vi "Client.vi"() -> ()   [LabVIEW 2020]
panel:
  out "Current Time":timestamp
  out "Login":bool
  in  "Tab Control":T1(tab)
  out "Status Word":string
  out "Status":bool
  in  "4":bool
  out "Pin Number":string
  in  "E":bool
  in  "0":bool
  in  "C":bool
  in  "9":bool
  in  "8":bool
  in  "7":bool
  in  "6":bool
  in  "5":bool
  in  "3":bool
  in  "2":bool
  in  "1":bool
  in  "Alarm System":bool
  in  "Door Automatically Open":bool
  in  "Holiday Mode":bool
  in  "Temperature(°C)":dbl(slide) scale=-20.0..50.0
  out "Temperature(°C)":dbl
  in  "Clock":timestamp
  in  "Master Curtain":bool
  in  "Master Door":bool
  in  "Master Light":bool
  in  "Living Area AirCon":bool
  in  "Brightness\n Porch Light":dbl(slide) scale=0.0..255.0
  in  "Brightness\nLiving Area Light 1":dbl(slide) scale=0.0..255.0
  in  "Brightness\nLiving Area Light 2":dbl(slide) scale=0.0..255.0
  in  "Porch Light":bool
  in  "Living Area Curtain":dbl(slide) scale=0.0..100.0
  in  "Main Door":bool
  in  "Volume":i32(knob) scale=0.0..100.0
  in  "Mute":bool
  in  "Fast Forward":bool
  in  "Fast Reverse":bool
  in  "Stop":bool
  in  "Pause":bool
  in  "Play":bool
  in  "On/Off":bool
  in  "Channel 2":bool
  in  "Channel 1":bool
  in  "Channel 3":bool
  in  "Channel 4":bool
  in  "Living Area Light 2":bool
  in  "Living Area Light 1":bool
  in  "Brightness\nLanai Light":dbl(slide) scale=0.0..255.0
  in  "Brightness\nDining Area Light 1":dbl(slide) scale=0.0..255.0
  in  "Brightness\nDining Area Light 2":dbl(slide) scale=0.0..255.0
  in  "Lanai Light":bool
  in  "Lanai Door":bool
  in  "Dining Area Light 2":bool
  in  "Dining Area Light 1":bool
  in  "Master Bedroom AirCon":bool
  in  "Brightness\nMaster Bedroom \nLight 1":dbl(slide) scale=0.0..255.0
  in  "Brightness\nMaster Bath \nLight":dbl(slide) scale=0.0..255.0
  in  "Brightness\nMaster Bedroom \nLight 2":dbl(slide) scale=0.0..255.0
  in  "Brightness\nMaster Bedroom \nW.I.C. Light":dbl(slide) scale=0.0..255.0
  in  "Master Bedroom Curtain":dbl(slide) scale=0.0..100.0
  in  "Master Bath Door":bool
  in  "Master Bedroom Door":bool
  in  "Master Bedroom W.I.C. Light":bool
  in  "Master Bath Light":bool
  in  "Master Bedroom Light 2":bool
  in  "Master Bedroom Light 1":bool
  in  "Bedroom 2 AirCon":bool
  in  "Brightness\nBedroom 2 \nLight 1":dbl(slide) scale=0.0..255.0
  in  "Brightness\nBedroom 2 \nLight 2":dbl(slide) scale=0.0..255.0
  in  "Brightness\nBedroom 2 \nW.I.C. Light":dbl(slide) scale=0.0..255.0
  in  "Bedroom 2 Curtain 2":dbl(slide) scale=0.0..100.0
  in  "Bedroom 2 Curtain 1":dbl(slide) scale=0.0..100.0
  in  "Bedroom 2 Door":bool
  in  "Bedroom 2 W.I.C. Light":bool
  in  "Bedroom 2 Light 2":bool
  in  "Bedroom 2 Light 1":bool
  in  "Bedroom 3 AirCon":bool
  in  "Brightness\nBedroom 3 \nLight 1":dbl(slide) scale=0.0..255.0
  in  "Brightness\nBedroom 3 \nLight 2":dbl(slide) scale=0.0..255.0
  in  "Bedroom 3 Curtain 2":dbl(slide) scale=0.0..100.0
  in  "Bedroom 3 Curtain 1":dbl(slide) scale=0.0..100.0
  in  "Bedroom 3 Door":bool
  in  "Bedroom 3 Light 2":bool
  in  "Bedroom 3 Light 1":bool
  in  "Brightness\nService Laundry \nLight 2":dbl(slide) scale=0.0..255.0
  in  "Brightness\nService Laundry \nLight 1":dbl(slide) scale=0.0..255.0
  in  "Service Laundry Light 1":bool
  in  "Service Laundry Light 2":bool
  in  "Service/Laundry Door":bool
  in  "Brightness\nT&B Light":dbl(slide) scale=0.0..255.0
  in  "Brightness\nKitchen \nLight 2":dbl(slide) scale=0.0..255.0
  in  "Brightness\nKitchen \nLight 1":dbl(slide) scale=0.0..255.0
  in  "Kitchen Curtain 2":dbl(slide) scale=0.0..100.0
  in  "Kitchen Curtain 1":dbl(slide) scale=0.0..100.0
  in  "T&B Door":bool
  in  "T&B Light":bool
  in  "Kitchen Light 2":bool
  in  "Kitchen Light 1":bool
  in  "Brightness\nGarage Light 1":dbl(slide) scale=0.0..255.0
  in  "Brightness\nGarage Light 2":dbl(slide) scale=0.0..255.0
  in  "Garage Light 2":bool
  in  "Garage Light 1":bool
  in  "Logout":bool
  # "Smart Home Control System"
  # "LOGIN PAGE"
  # "Main Control"
  # "Living Area"
  # "TV"
  # "Dining Area"
  # "Lanai"
  # "Lanai"
  # "Master Bedroom"
  # "Bedroom 2"
  # "Bedroom 3"
  # "Kitchen"
  # "Service / Laundry"
  # "Garage"
  # "Are you sure want to logout?"
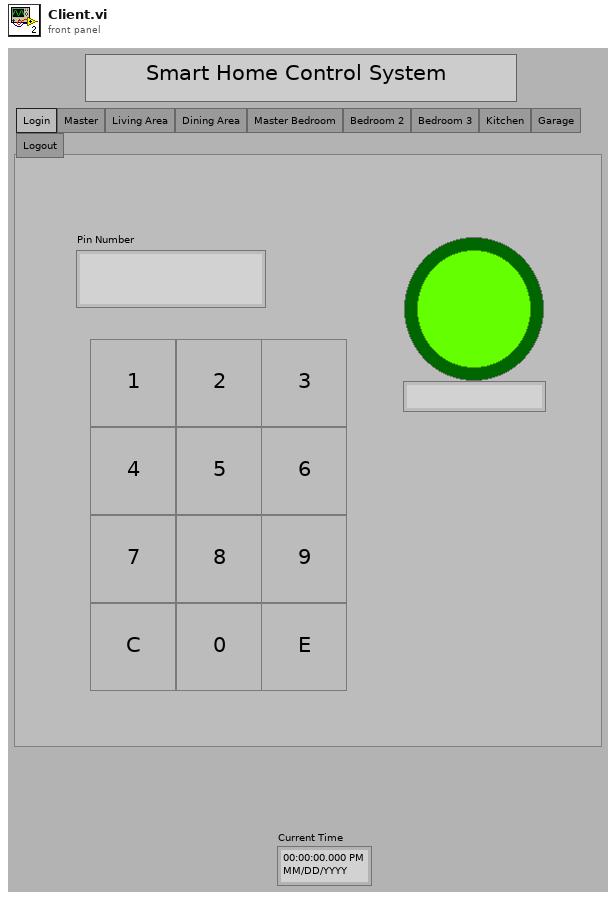
[diagram p1: front panel]
types:
  T1 = enum32{"Login", "Master", "Living Area", "Dining Area", "Master Bedroom", "Bedroom 2", "Bedroom 3", "Kitchen", "Garage", "Logout"}
  T2 = enum32{"Page Enabled", "Page Disabled", "Page Disabled & Grayed"}
  T3 = enum32{"Invalid", "Standard", "Closed", "Hidden", "Minimized", "Maximized"}
  T4 = typedef "LVDateTimeRec.ctl" = cluster{"fractional second":dbl, "second":i32, "minute":i32, "hour":i32, "day of month":i32, "month":i32, "year":i32, "day of week":i32, "day of year":i32, "DST":i32}
  T5 = enum8{"Enabled", "Disabled", "Disabled and Grayed Out"}
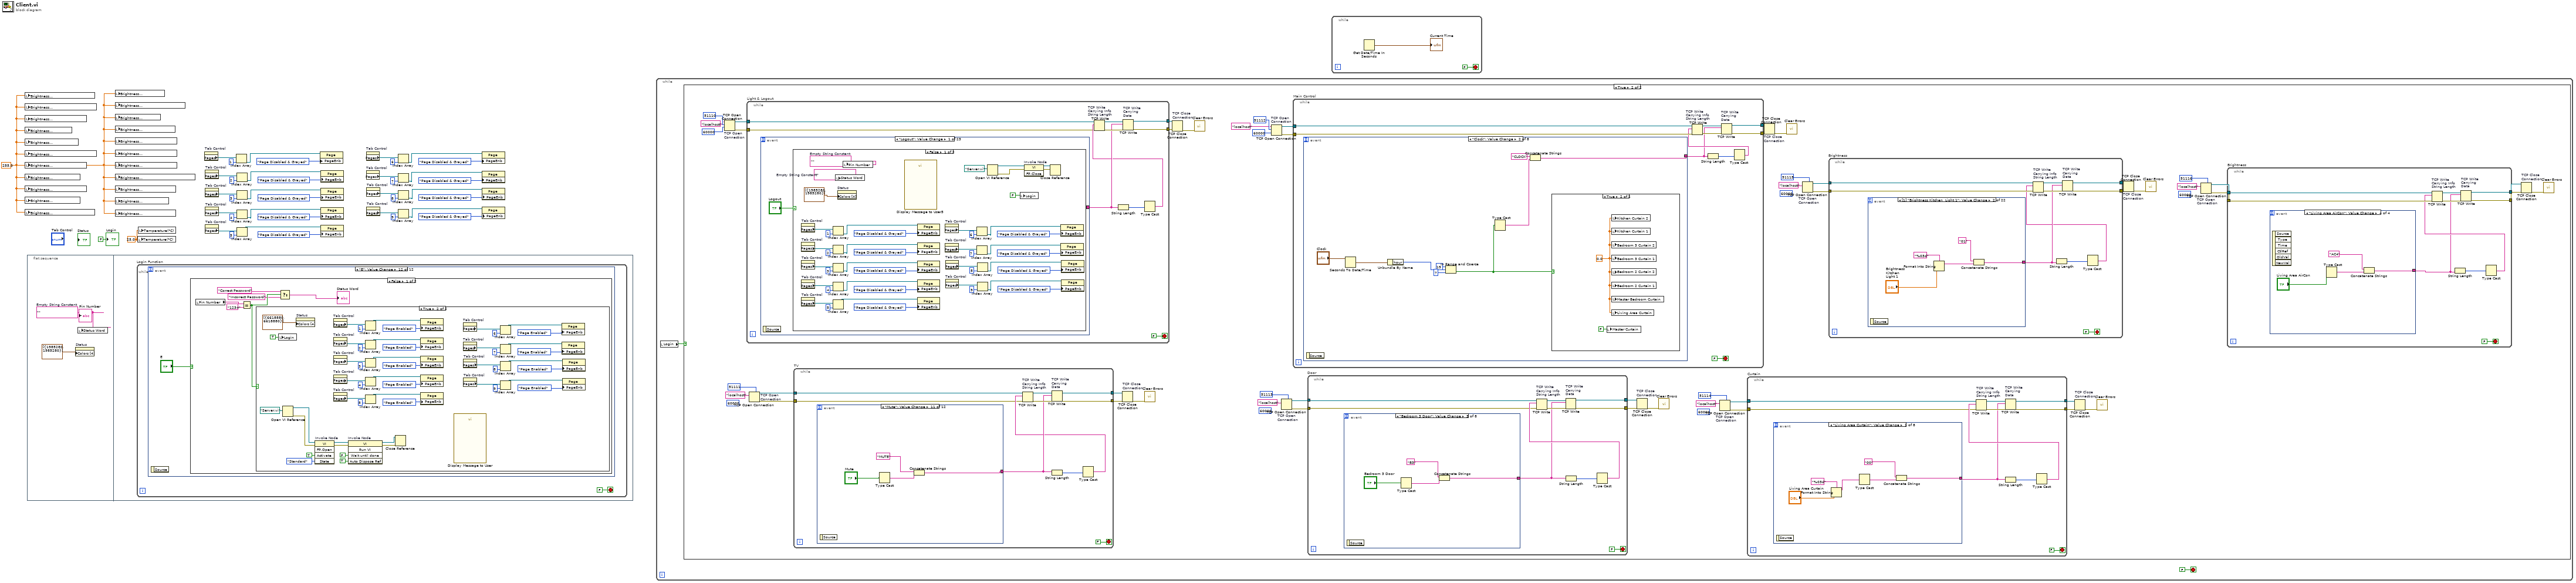
[diagram p0: block diagram]
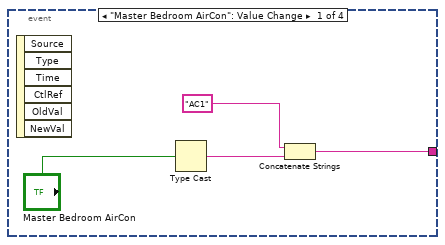
[diagram p3: hidden frame]
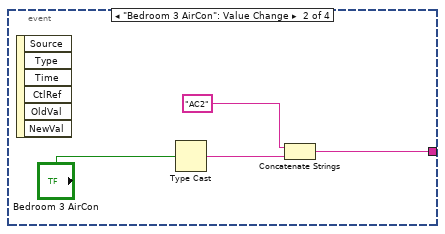
[diagram p4: hidden frame]
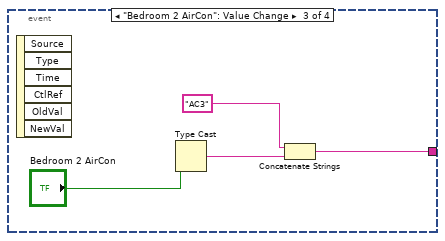
[diagram p5: hidden frame]
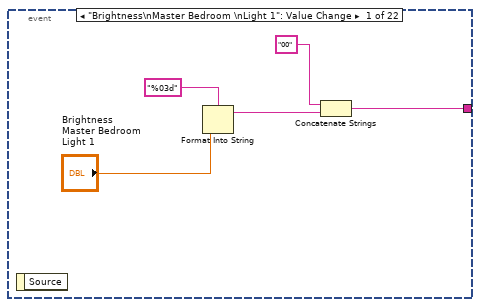
[diagram p6: hidden frame]
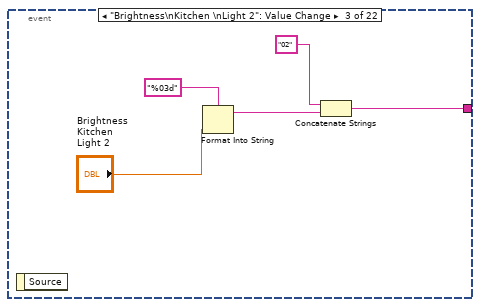
[diagram p7: hidden frame]
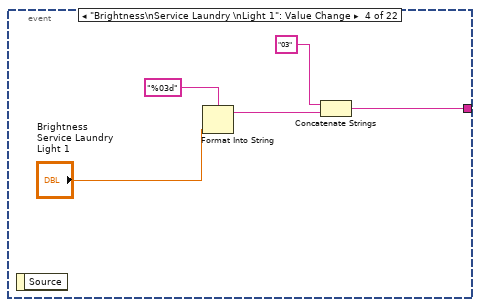
[diagram p8: hidden frame]
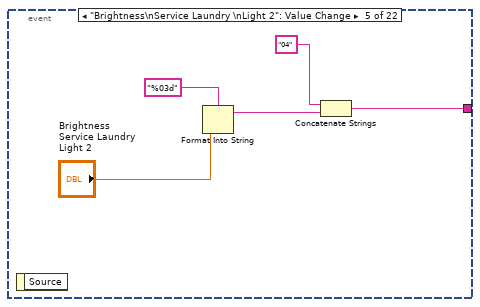
[diagram p9: hidden frame]
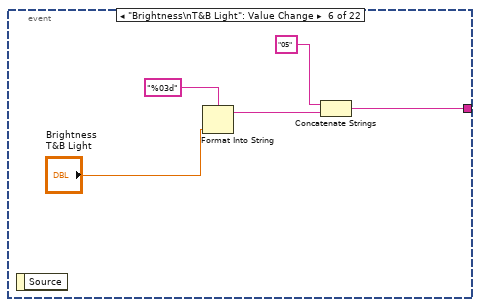
[diagram p10: hidden frame]
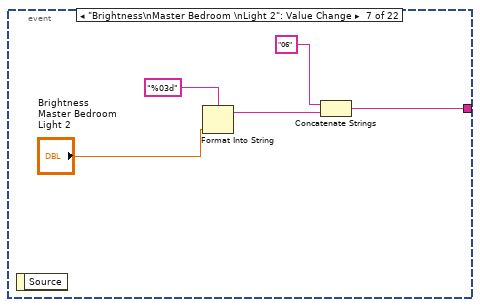
[diagram p11: hidden frame]
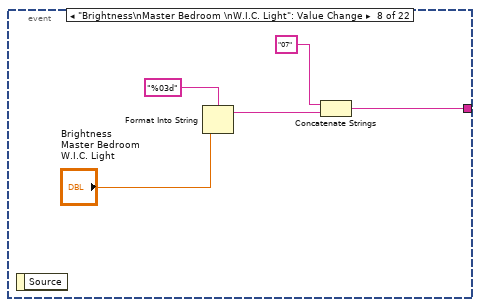
[diagram p12: hidden frame]
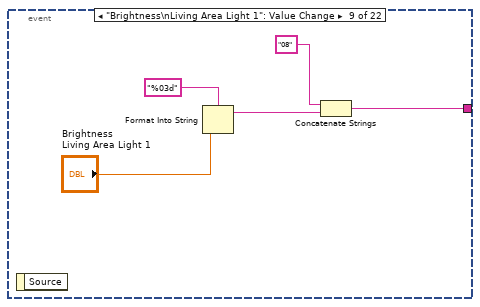
[diagram p13: hidden frame]
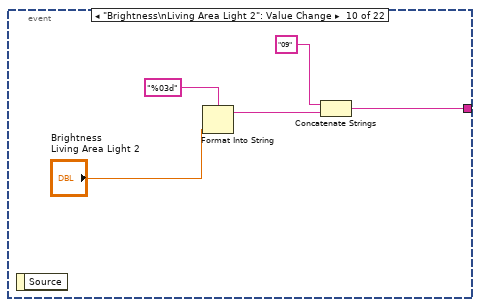
[diagram p14: hidden frame]
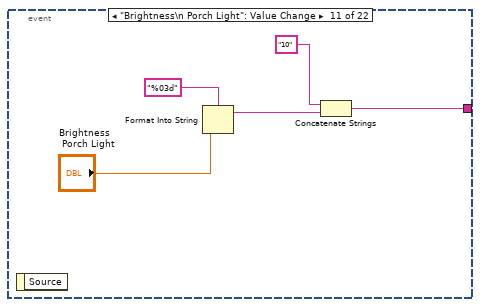
[diagram p15: hidden frame]
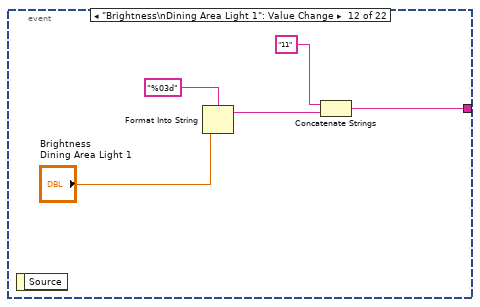
[diagram p16: hidden frame]
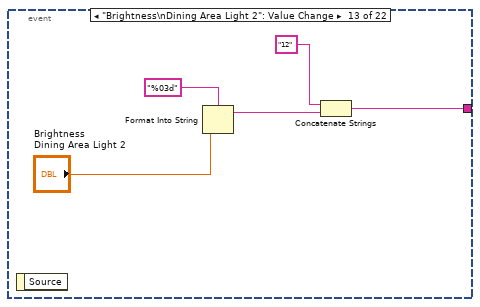
[diagram p17: hidden frame]
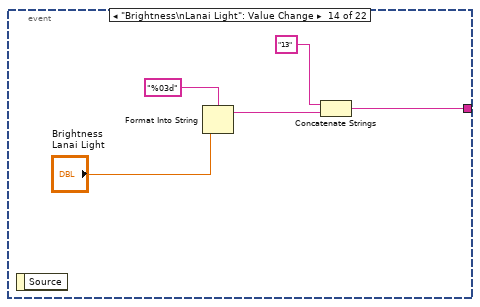
[diagram p18: hidden frame]
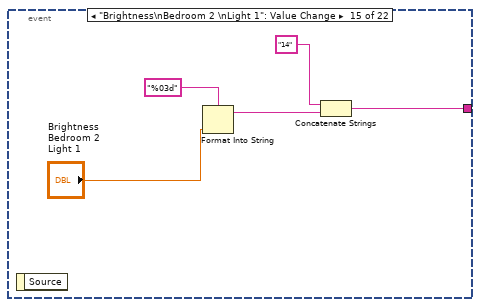
[diagram p19: hidden frame]
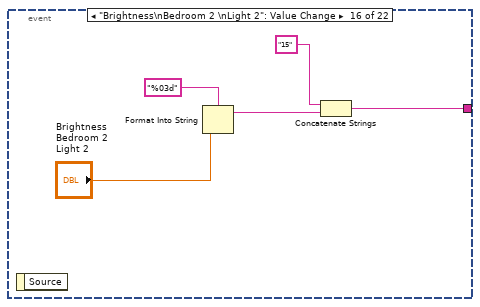
[diagram p20: hidden frame]
diagram:
  w1 = 255.0 ("Brightness\nBedroom 2 \nLight 1")
  w38 = 25.0 ("Temperature(°C)")
  n1 = local write "Brightness\nService Laundry \nLight 2"(w1) -> ()
  n2 = local write "Brightness\nMaster Bedroom \nLight 2"(w1) -> ()
  n3 = local write "Brightness\nDining Area Light 2"(w1) -> ()
  n4 = local write "Brightness\nLanai Light"(w1) -> ()
  n5 = local write "Brightness\nGarage Light 2"(w1) -> ()
  n6 = local write "Brightness\nMaster Bedroom \nLight 1"(w1) -> ()
  n7 = local write "Brightness\nBedroom 2 \nLight 1"(w1) -> ()
  n8 = local write "Brightness\nKitchen \nLight 1"(w1) -> ()
  n9 = local write "Brightness\nBedroom 2 \nLight 2"(w1) -> ()
  n10 = local write "Brightness\nKitchen \nLight 2"(w1) -> ()
  n11 = local write "Brightness\nBedroom 2 \nW.I.C. Light"(w1) -> ()
  n12 = flat-sequence {
    frame #0 {
      w40 = ""  # Empty String Constant
      n13 = property on="Status" class="Bool (strict)"("Colors [4]"=cluster{u32, u32}[] [{1985280, 1985280}]) -> ()  [unwired: 2 in, 2 out]
      n14 = local write "Status Word"(w40) -> ()
      "Pin Number" <- w40
    }
    frame #1 {
      n15 = while "Login Function" {
        stop <- FALSE stop-if-true
        n16 = event shown="[11] \"E\": Value Change" {
          selector: _ -> [_ _ _ _ _ _ _ _ _ _ _ _]
          dyn-events: _ -> [_ _ _ _ _ _ _ _ _ _ _ _]
          timeout: _ -> [_ _ _ _ _ _ _ _ _ _ _ _]
          event "1": Value Change {
            n17 = event-data() -> ()  [unwired: 1 in, 1 out]
            n18 = case shown="False" "1" {
              frame False {
                n19 = local read "Pin Number"() -> (w47:string)
                n20 = String Length "String \nLength"(string=w47) -> (length=w46:i32)
                n21 = Less?(x=w46, y=4) -> (x < y?=w44:bool)
                n22 = case shown="True" w44 {
                  frame False {
                  }
                  frame True {
                    n23 = local read "Pin Number"() -> (w50:string)
                    n24 = Concatenate Strings "Concatenate \nStrings"(w50, "1" ("string")) -> (w49:string)
                    n25 = local write "Pin Number"(w49) -> ()
                  }
                }
              }
              frame True {
              }
            }
          }
          event "2": Value Change {
            n26 = event-data() -> ()  [unwired: 1 in, 1 out]
            n27 = case shown="False" "2" {
              frame False {
                n28 = local read "Pin Number"() -> (w55:string)
                n29 = String Length "String \nLength"(string=w55) -> (length=w54:i32)
                n30 = Less?(x=w54, y=4) -> (x < y?=w52:bool)
                n31 = case shown="True" w52 {
                  frame False {
                  }
                  frame True {
                    n32 = local read "Pin Number"() -> (w58:string)
                    n33 = Concatenate Strings "Concatenate \nStrings"(w58, "2" ("string")) -> (w57:string)
                    n34 = local write "Pin Number"(w57) -> ()
                  }
                }
              }
              frame True {
              }
            }
          }
          event "3": Value Change {
            n35 = event-data() -> ()  [unwired: 1 in, 1 out]
            n36 = case shown="False" "3" {
              frame False {
                n37 = local read "Pin Number"() -> (w63:string)
                n38 = String Length "String \nLength"(string=w63) -> (length=w62:i32)
                n39 = Less?(x=w62, y=4) -> (x < y?=w60:bool)
                n40 = case shown="True" w60 {
                  frame False {
                  }
                  frame True {
                    n41 = local read "Pin Number"() -> (w66:string)
                    n42 = Concatenate Strings "Concatenate \nStrings"(w66, "3" ("string")) -> (w65:string)
                    n43 = local write "Pin Number"(w65) -> ()
                  }
                }
              }
              frame True {
              }
            }
          }
          event "4": Value Change {
            n44 = event-data() -> ()  [unwired: 1 in, 1 out]
            n45 = case shown="False" "4" {
              frame False {
                n46 = local read "Pin Number"() -> (w71:string)
                n47 = String Length "String \nLength"(string=w71) -> (length=w70:i32)
                n48 = Less?(x=w70, y=4) -> (x < y?=w68:bool)
                n49 = case shown="True" w68 {
                  frame False {
                  }
                  frame True {
                    n50 = local read "Pin Number"() -> (w74:string)
                    n51 = Concatenate Strings "Concatenate \nStrings"(w74, "4" ("string")) -> (w73:string)
                    n52 = local write "Pin Number"(w73) -> ()
                  }
                }
              }
              frame True {
              }
            }
          }
          event "5": Value Change {
            n53 = event-data() -> ()  [unwired: 1 in, 1 out]
            n54 = case shown="False" "5" {
              frame False {
                n55 = local read "Pin Number"() -> (w79:string)
                n56 = String Length "String \nLength"(string=w79) -> (length=w78:i32)
                n57 = Less?(x=w78, y=4) -> (x < y?=w76:bool)
                n58 = case shown="True" w76 {
                  frame False {
                  }
                  frame True {
                    n59 = local read "Pin Number"() -> (w82:string)
                    n60 = Concatenate Strings "Concatenate \nStrings"(w82, "5" ("string")) -> (w81:string)
                    n61 = local write "Pin Number"(w81) -> ()
                  }
                }
              }
              frame True {
              }
            }
          }
          event "6": Value Change {
            n62 = event-data() -> ()  [unwired: 1 in, 1 out]
            n63 = case shown="False" "6" {
              frame False {
                n64 = local read "Pin Number"() -> (w87:string)
                n65 = String Length "String \nLength"(string=w87) -> (length=w86:i32)
                n66 = Less?(x=w86, y=4) -> (x < y?=w84:bool)
                n67 = case shown="True" w84 {
                  frame False {
                  }
                  frame True {
                    n68 = local read "Pin Number"() -> (w90:string)
                    n69 = Concatenate Strings "Concatenate \nStrings"(w90, "6" ("string")) -> (w89:string)
                    n70 = local write "Pin Number"(w89) -> ()
                  }
                }
              }
              frame True {
              }
            }
          }
          event "7": Value Change {
            n71 = event-data() -> ()  [unwired: 1 in, 1 out]
            n72 = case shown="False" "7" {
              frame False {
                n73 = local read "Pin Number"() -> (w95:string)
                n74 = String Length "String \nLength"(string=w95) -> (length=w94:i32)
                n75 = Less?(x=w94, y=4) -> (x < y?=w92:bool)
                n76 = case shown="True" w92 {
                  frame False {
                  }
                  frame True {
                    n77 = local read "Pin Number"() -> (w98:string)
                    n78 = Concatenate Strings "Concatenate \nStrings"(w98, "7" ("string")) -> (w97:string)
                    n79 = local write "Pin Number"(w97) -> ()
                  }
                }
              }
              frame True {
              }
            }
          }
          event "8": Value Change {
            n80 = event-data() -> ()  [unwired: 1 in, 1 out]
            n81 = case shown="False" "8" {
              frame False {
                n82 = local read "Pin Number"() -> (w103:string)
                n83 = String Length "String \nLength"(string=w103) -> (length=w102:i32)
                n84 = Less?(x=w102, y=4) -> (x < y?=w100:bool)
                n85 = case shown="True" w100 {
                  frame False {
                  }
                  frame True {
                    n86 = local read "Pin Number"() -> (w106:string)
                    n87 = Concatenate Strings "Concatenate \nStrings"(w106, "8" ("string")) -> (w105:string)
                    n88 = local write "Pin Number"(w105) -> ()
                  }
                }
              }
              frame True {
              }
            }
          }
          event "9": Value Change {
            n89 = event-data() -> ()  [unwired: 1 in, 1 out]
            n90 = case shown="False" "9" {
              frame False {
                n91 = local read "Pin Number"() -> (w111:string)
                n92 = String Length "String \nLength"(string=w111) -> (length=w110:i32)
                n93 = Less?(x=w110, y=4) -> (x < y?=w108:bool)
                n94 = case shown="True" w108 {
                  frame False {
                  }
                  frame True {
                    n95 = local read "Pin Number"() -> (w114:string)
                    n96 = Concatenate Strings "Concatenate \nStrings"(w114, "9" ("string")) -> (w113:string)
                    n97 = local write "Pin Number"(w113) -> ()
                  }
                }
              }
              frame True {
              }
            }
          }
          event "0": Value Change {
            n98 = event-data() -> ()  [unwired: 1 in, 1 out]
            n99 = case shown="False" "0" {
              frame False {
                n100 = local read "Pin Number"() -> (w119:string)
                n101 = String Length "String \nLength"(string=w119) -> (length=w118:i32)
                n102 = Less?(x=w118, y=4) -> (x < y?=w116:bool)
                n103 = case shown="True" w116 {
                  frame False {
                  }
                  frame True {
                    n104 = local read "Pin Number"() -> (w122:string)
                    n105 = Concatenate Strings "Concatenate \nStrings"(w122, "0" ("string")) -> (w121:string)
                    n106 = local write "Pin Number"(w121) -> ()
                  }
                }
              }
              frame True {
              }
            }
          }
          event "C": Value Change {
            n107 = event-data() -> ()  [unwired: 1 in, 1 out]
            n108 = case shown="False" "C" {
              frame False {
                w124 = ""  # Empty String Constant
                n109 = local write "Pin Number"(w124) -> ()
              }
              frame True {
              }
            }
          }
          event "E": Value Change {
            n110 = event-data() -> ()  [unwired: 1 in, 1 out]
            n111 = case shown="False" "E" {
              frame False {
                n112 = local read "Pin Number"() -> (w131:string)
                n113 = Equal?(x=w131, y="1234") -> (x = y?=w129:bool)
                n114 = case shown="True" w129 {
                  frame False {
                    n115 = property on="Status" class="Bool (strict)"("Colors [4]"=cluster{u32, u32}[] [{16713728, 16714752}]) -> ()  [unwired: 2 in, 2 out]
                  }
                  frame True {
                    n116 = local write "Login"(TRUE ("Login")) -> ()
                    n117 = Open VI Reference(vi path=path "Server.vi") -> (vi reference=w179:refnum<vi>, error out=w178:errorcluster)  [unwired: 5 in]
                    n118 = property on="Status" class="Bool (strict)"("Colors [4]"=cluster{u32, u32}[] [{6618880, 6618880}]) -> ()  [unwired: 2 in, 2 out]
                    n119 = invoke on="Invoke Node" class="VI" method="FP.Open"(reference=w179, error in=w178, "Activate"=TRUE ("Activate?"), "State"=T3."Standard") -> (reference out=w173:refnum<vi>, error out=w172:errorcluster)  [unwired: 1 in, 3 out]
                    n120 = property on="Tab Control" class="TabCtl (strict)"() -> ("Pages"=w163:refnum<vi>[])  [unwired: 2 in, 2 out]
                    n121 = property on="Tab Control" class="TabCtl (strict)"() -> ("Pages"=w158:refnum<vi>[])  [unwired: 2 in, 2 out]
                    n122 = property on="Tab Control" class="TabCtl (strict)"() -> ("Pages"=w150:refnum<vi>[])  [unwired: 2 in, 2 out]
                    n123 = property on="Tab Control" class="TabCtl (strict)"() -> ("Pages"=w155:refnum<vi>[])  [unwired: 2 in, 2 out]
                    n124 = property on="Tab Control" class="TabCtl (strict)"() -> ("Pages"=w166:refnum<vi>[])  [unwired: 2 in, 2 out]
                    n125 = invoke on="Invoke Node" class="VI" method="Run VI"(reference=w173, error in=w172, "Wait until done"=FALSE ("Wait Until Done"), "Auto Dispose Ref"=TRUE ("Auto Dispose Reference")) -> (reference out=w171:refnum<vi>, error out=w170:errorcluster)  [unwired: 1 in, 3 out]
                    n126 = Index Array "Index Array"(array=w163, index=1) -> (element=w162:refnum<vi>)
                    n127 = Index Array "Index Array"(array=w158, index=2) -> (element=w159:refnum<vi>)
                    n128 = Index Array "Index Array"(array=w150, index=3) -> (element=w151:refnum<vi>)
                    n129 = Index Array "Index Array"(array=w155, index=4) -> (element=w154:refnum<vi>)
                    n130 = Index Array "Index Array"(array=w166, index=5) -> (element=w168:refnum<vi>)
                    n131 = Close Reference(reference=w171, error in (no error)=w170) -> ()  [unwired: 1 out]
                    n132 = property class="Page"(reference=w162, "PageEnb"=T2."Page Enabled" ("Page Enabled State")) -> ()  [unwired: 1 in, 2 out]
                    n133 = property class="Page"(reference=w159, "PageEnb"=T2."Page Enabled" ("Page Enabled State")) -> ()  [unwired: 1 in, 2 out]
                    n134 = property class="Page"(reference=w151, "PageEnb"=T2."Page Enabled" ("Page Enabled State")) -> ()  [unwired: 1 in, 2 out]
                    n135 = property class="Page"(reference=w154, "PageEnb"=T2."Page Enabled" ("Page Enabled State")) -> ()  [unwired: 1 in, 2 out]
                    n136 = property class="Page"(reference=w168, "PageEnb"=T2."Page Enabled" ("Page Enabled State")) -> ()  [unwired: 1 in, 2 out]
                    n137 = call "Display Message to User"() -> ()  [unwired: 10 in, 2 out]
                    n138 = property on="Tab Control" class="TabCtl (strict)"() -> ("Pages"=w141:refnum<vi>[])  [unwired: 2 in, 2 out]
                    n139 = property on="Tab Control" class="TabCtl (strict)"() -> ("Pages"=w144:refnum<vi>[])  [unwired: 2 in, 2 out]
                    n140 = property on="Tab Control" class="TabCtl (strict)"() -> ("Pages"=w148:refnum<vi>[])  [unwired: 2 in, 2 out]
                    n141 = property on="Tab Control" class="TabCtl (strict)"() -> ("Pages"=w145:refnum<vi>[])  [unwired: 2 in, 2 out]
                    n142 = Index Array "Index Array"(array=w141, index=6) -> (element=w142:refnum<vi>)
                    n143 = Index Array "Index Array"(array=w144, index=7) -> (element=w143:refnum<vi>)
                    n144 = Index Array "Index Array"(array=w148, index=8) -> (element=w147:refnum<vi>)
                    n145 = Index Array "Index Array"(array=w145, index=9) -> (element=w146:refnum<vi>)
                    n146 = property class="Page"(reference=w142, "PageEnb"=T2."Page Enabled" ("Page Enabled State")) -> ()  [unwired: 1 in, 2 out]
                    n147 = property class="Page"(reference=w143, "PageEnb"=T2."Page Enabled" ("Page Enabled State")) -> ()  [unwired: 1 in, 2 out]
                    n148 = property class="Page"(reference=w147, "PageEnb"=T2."Page Enabled" ("Page Enabled State")) -> ()  [unwired: 1 in, 2 out]
                    n149 = property class="Page"(reference=w146, "PageEnb"=T2."Page Enabled" ("Page Enabled State")) -> ()  [unwired: 1 in, 2 out]
                  }
                }
                n150 = Select(t="Correct Password", s=w129, f="Incorrect Password") -> (s? t:f=→"Status Word":string)
              }
              frame True {
              }
            }
          }
        }
      }
    }
  }
  n151 = local write "Brightness\n Porch Light"(w1) -> ()
  n152 = local write "Brightness\nService Laundry \nLight 1"(w1) -> ()
  n153 = local write "Brightness\nT&B Light"(w1) -> ()
  n154 = local write "Brightness\nMaster Bath \nLight"(w1) -> ()
  n155 = local write "Brightness\nDining Area Light 1"(w1) -> ()
  n156 = local write "Brightness\nBedroom 3 \nLight 1"(w1) -> ()
  n157 = local write "Brightness\nBedroom 3 \nLight 2"(w1) -> ()
  n158 = local write "Brightness\nMaster Bedroom \nW.I.C. Light"(w1) -> ()
  n159 = local write "Brightness\nLiving Area Light 1"(w1) -> ()
  n160 = local write "Brightness\nGarage Light 1"(w1) -> ()
  n161 = local write "Brightness\nLiving Area Light 2"(w1) -> ()
  n162 = local write "Temperature(°C)"(w38) -> ()
  n163 = local write "Temperature(°C)"(w38) -> ()
  n164 = property on="Tab Control" class="TabCtl (strict)"() -> ("Pages"=w7:refnum<vi>[])  [unwired: 2 in, 2 out]
  n165 = property on="Tab Control" class="TabCtl (strict)"() -> ("Pages"=w12:refnum<vi>[])  [unwired: 2 in, 2 out]
  n166 = property on="Tab Control" class="TabCtl (strict)"() -> ("Pages"=w20:refnum<vi>[])  [unwired: 2 in, 2 out]
  n167 = property on="Tab Control" class="TabCtl (strict)"() -> ("Pages"=w15:refnum<vi>[])  [unwired: 2 in, 2 out]
  n168 = property on="Tab Control" class="TabCtl (strict)"() -> ("Pages"=w4:refnum<vi>[])  [unwired: 2 in, 2 out]
  n169 = Index Array "Index Array"(array=w7, index=1) -> (element=w8:refnum<vi>)
  n170 = Index Array "Index Array"(array=w12, index=2) -> (element=w11:refnum<vi>)
  n171 = Index Array "Index Array"(array=w20, index=3) -> (element=w19:refnum<vi>)
  n172 = Index Array "Index Array"(array=w15, index=4) -> (element=w16:refnum<vi>)
  n173 = Index Array "Index Array"(array=w4, index=5) -> (element=w2:refnum<vi>)
  n174 = property class="Page"(reference=w8, "PageEnb"=T2."Page Disabled & Grayed" ("Page Enabled State")) -> ()  [unwired: 1 in, 2 out]
  n175 = property class="Page"(reference=w11, "PageEnb"=T2."Page Disabled & Grayed" ("Page Enabled State")) -> ()  [unwired: 1 in, 2 out]
  n176 = property class="Page"(reference=w19, "PageEnb"=T2."Page Disabled & Grayed" ("Page Enabled State")) -> ()  [unwired: 1 in, 2 out]
  n177 = property class="Page"(reference=w16, "PageEnb"=T2."Page Disabled & Grayed" ("Page Enabled State")) -> ()  [unwired: 1 in, 2 out]
  n178 = property class="Page"(reference=w2, "PageEnb"=T2."Page Disabled & Grayed" ("Page Enabled State")) -> ()  [unwired: 1 in, 2 out]
  n179 = property on="Tab Control" class="TabCtl (strict)"() -> ("Pages"=w36:refnum<vi>[])  [unwired: 2 in, 2 out]
  n180 = property on="Tab Control" class="TabCtl (strict)"() -> ("Pages"=w31:refnum<vi>[])  [unwired: 2 in, 2 out]
  n181 = property on="Tab Control" class="TabCtl (strict)"() -> ("Pages"=w23:refnum<vi>[])  [unwired: 2 in, 2 out]
  n182 = property on="Tab Control" class="TabCtl (strict)"() -> ("Pages"=w28:refnum<vi>[])  [unwired: 2 in, 2 out]
  n183 = Index Array "Index Array"(array=w36, index=6) -> (element=w35:refnum<vi>)
  n184 = Index Array "Index Array"(array=w31, index=7) -> (element=w32:refnum<vi>)
  n185 = Index Array "Index Array"(array=w23, index=8) -> (element=w24:refnum<vi>)
  n186 = Index Array "Index Array"(array=w28, index=9) -> (element=w27:refnum<vi>)
  n187 = property class="Page"(reference=w35, "PageEnb"=T2."Page Disabled & Grayed" ("Page Enabled State")) -> ()  [unwired: 1 in, 2 out]
  n188 = property class="Page"(reference=w32, "PageEnb"=T2."Page Disabled & Grayed" ("Page Enabled State")) -> ()  [unwired: 1 in, 2 out]
  n189 = property class="Page"(reference=w24, "PageEnb"=T2."Page Disabled & Grayed" ("Page Enabled State")) -> ()  [unwired: 1 in, 2 out]
  n190 = property class="Page"(reference=w27, "PageEnb"=T2."Page Disabled & Grayed" ("Page Enabled State")) -> ()  [unwired: 1 in, 2 out]
  n191 = while {
    stop <- FALSE stop-if-true
    n192 = local read "Login"() -> (w183:bool)
    n193 = case shown="True" w183 {
      frame False {
      }
      frame True {
        (unwired) 60000 ("timeout ms (60000)")
        (unwired) 60000 ("timeout ms (60000)")
        (unwired) 60000 ("timeout ms (60000)")
        (unwired) 60000 ("timeout ms (60000)")
        (unwired) 60000 ("timeout ms (60000)")
        n194 = TCP Open Connection "TCP Open \nConnection"(address="localhost", remote port or service name=u16 51110, timeout ms (60000)=60000) -> (connection ID=w230:refnum<k5>, error out=w231:errorcluster)  [unwired: 2 in]
        n195 = while "Light & Logout" {
          tunnel: w231 -> [w614]
          tunnel: w230 -> [w613]
          tunnel: [w612] -> w228
          tunnel: [w611] -> w227
          stop <- FALSE stop-if-true
          n196 = event shown="[0] \"Logout\": Value Change" {
            selector: _ -> [_ _ _ _ _ _ _ _ _ _ _ _ _ _ _ _ _ _ _ _ _ _ _]
            dyn-events: _ -> [_ _ _ _ _ _ _ _ _ _ _ _ _ _ _ _ _ _ _ _ _ _ _]
            timeout: _ -> [_ _ _ _ _ _ _ _ _ _ _ _ _ _ _ _ _ _ _ _ _ _ _]
            tunnel: [_ w666 w671 w675 w679 w683 w687 w691 w695 w699 w703 w707 w711 w715 w719 w723 w727 w731 w735 w739 w743 w747 w751] -> w617
            event "Logout": Value Change {
              n197 = event-data() -> ()  [unwired: 1 in, 1 out]
              n198 = case shown="False" "Logout" {
                frame False {
                  w659 = ""  # Empty String Constant
                  w657 = ""  # Empty String Constant
                  n199 = property on="Tab Control" class="TabCtl (strict)"() -> ("Pages"=w641:refnum<vi>[])  [unwired: 2 in, 2 out]
                  n200 = property on="Tab Control" class="TabCtl (strict)"() -> ("Pages"=w644:refnum<vi>[])  [unwired: 2 in, 2 out]
                  n201 = property on="Tab Control" class="TabCtl (strict)"() -> ("Pages"=w648:refnum<vi>[])  [unwired: 2 in, 2 out]
                  n202 = property on="Tab Control" class="TabCtl (strict)"() -> ("Pages"=w645:refnum<vi>[])  [unwired: 2 in, 2 out]
                  n203 = property on="Tab Control" class="TabCtl (strict)"() -> ("Pages"=w640:refnum<vi>[])  [unwired: 2 in, 2 out]
                  n204 = Index Array "Index Array"(array=w641, index=1) -> (element=w642:refnum<vi>)
                  n205 = Index Array "Index Array"(array=w644, index=2) -> (element=w643:refnum<vi>)
                  n206 = Index Array "Index Array"(array=w648, index=3) -> (element=w647:refnum<vi>)
                  n207 = Index Array "Index Array"(array=w645, index=4) -> (element=w646:refnum<vi>)
                  n208 = Index Array "Index Array"(array=w640, index=5) -> (element=w639:refnum<vi>)
                  n209 = local write "Status Word"(w657) -> ()
                  n210 = property on="Status" class="Bool (strict)"("Colors [4]"=cluster{u32, u32}[] [{1985280, 1985280}]) -> ()  [unwired: 2 in, 2 out]
                  n211 = local write "Pin Number"(w659) -> ()
                  n212 = call "Display Message to User3"() -> ()  [unwired: 10 in, 2 out]
                  n213 = property class="Page"(reference=w642, "PageEnb"=T2."Page Disabled & Grayed" ("Page Enabled State")) -> ()  [unwired: 1 in, 2 out]
                  n214 = property class="Page"(reference=w643, "PageEnb"=T2."Page Disabled & Grayed" ("Page Enabled State")) -> ()  [unwired: 1 in, 2 out]
                  n215 = property class="Page"(reference=w647, "PageEnb"=T2."Page Disabled & Grayed" ("Page Enabled State")) -> ()  [unwired: 1 in, 2 out]
                  n216 = property class="Page"(reference=w646, "PageEnb"=T2."Page Disabled & Grayed" ("Page Enabled State")) -> ()  [unwired: 1 in, 2 out]
                  n217 = property class="Page"(reference=w639, "PageEnb"=T2."Page Disabled & Grayed" ("Page Enabled State")) -> ()  [unwired: 1 in, 2 out]
                  n218 = property on="Tab Control" class="TabCtl (strict)"() -> ("Pages"=w656:refnum<vi>[])  [unwired: 2 in, 2 out]
                  n219 = property on="Tab Control" class="TabCtl (strict)"() -> ("Pages"=w653:refnum<vi>[])  [unwired: 2 in, 2 out]
                  n220 = property on="Tab Control" class="TabCtl (strict)"() -> ("Pages"=w649:refnum<vi>[])  [unwired: 2 in, 2 out]
                  n221 = property on="Tab Control" class="TabCtl (strict)"() -> ("Pages"=w652:refnum<vi>[])  [unwired: 2 in, 2 out]
                  n222 = Index Array "Index Array"(array=w656, index=6) -> (element=w655:refnum<vi>)
                  n223 = Index Array "Index Array"(array=w653, index=7) -> (element=w654:refnum<vi>)
                  n224 = Index Array "Index Array"(array=w649, index=8) -> (element=w650:refnum<vi>)
                  n225 = Index Array "Index Array"(array=w652, index=9) -> (element=w651:refnum<vi>)
                  n226 = Open VI Reference(vi path=path "Server.vi") -> (vi reference=w664:refnum<vi>, error out=w665:errorcluster)  [unwired: 5 in]
                  n227 = local write "Login"(FALSE ("Status 2")) -> ()
                  n228 = invoke on="Invoke Node" class="VI" method="FP.Close"(reference=w664, error in=w665) -> (reference out=w663:refnum<vi>, error out=w662:errorcluster)  [unwired: 1 in, 1 out]
                  n229 = Close Reference(reference=w663, error in (no error)=w662) -> ()  [unwired: 1 out]
                  n230 = property class="Page"(reference=w655, "PageEnb"=T2."Page Disabled & Grayed" ("Page Enabled State")) -> ()  [unwired: 1 in, 2 out]
                  n231 = property class="Page"(reference=w654, "PageEnb"=T2."Page Disabled & Grayed" ("Page Enabled State")) -> ()  [unwired: 1 in, 2 out]
                  n232 = property class="Page"(reference=w650, "PageEnb"=T2."Page Disabled & Grayed" ("Page Enabled State")) -> ()  [unwired: 1 in, 2 out]
                  n233 = property class="Page"(reference=w651, "PageEnb"=T2."Page Disabled & Grayed" ("Page Enabled State")) -> ()  [unwired: 1 in, 2 out]
                }
                frame True {
                }
              }
            }
            event "Porch Light": Value Change {
              n234 = event-data() -> ()  [unwired: 1 in, 1 out]
              n235 = case shown="True" "Porch Light" {
                tunnel: ["PL/F" "PL/T"] -> w666
                frame False {
                }
                frame True {
                }
              }
            }
            event "Living Area Light 1": Value Change {
              n236 = event-data() -> ()  [unwired: 1 in, 1 out]
              n237 = case shown="True" "Living Area Light 1" {
                tunnel: ["LAL1/F" "LAL1/T"] -> w671
                frame False {
                }
                frame True {
                }
              }
            }
            event "Living Area Light 2": Value Change {
              n238 = event-data() -> ()  [unwired: 1 in, 1 out]
              n239 = case shown="True" "Living Area Light 2" {
                tunnel: ["LAL2/F" "LAL2/T"] -> w675
                frame False {
                }
                frame True {
                }
              }
            }
            event "Dining Area Light 1": Value Change {
              n240 = event-data() -> ()  [unwired: 1 in, 1 out]
              n241 = case shown="True" "Dining Area Light 1" {
                tunnel: ["DAL1/F" "DAL1/T"] -> w679
                frame False {
                }
                frame True {
                }
              }
            }
            event "Dining Area Light 2": Value Change {
              n242 = event-data() -> ()  [unwired: 1 in, 1 out]
              n243 = case shown="True" "Dining Area Light 2" {
                tunnel: ["DAL2/F" "DAL2/T"] -> w683
                frame False {
                }
                frame True {
                }
              }
            }
            event "Master Bedroom Light 1": Value Change {
              n244 = event-data() -> ()  [unwired: 1 in, 1 out]
              n245 = case shown="False" "Master Bedroom Light 1" {
                tunnel: ["MBL1/F" "MBL1/T"] -> w687
                frame False {
                }
                frame True {
                }
              }
            }
            event "Master Bedroom Light 2": Value Change {
              n246 = event-data() -> ()  [unwired: 1 in, 1 out]
              n247 = case shown="False" "Master Bedroom Light 2" {
                tunnel: ["MBL2/F" "MBL2/T"] -> w691
                frame False {
                }
                frame True {
                }
              }
            }
            event "Master Bath Light": Value Change {
              n248 = event-data() -> ()  [unwired: 1 in, 1 out]
              n249 = case shown="True" "Master Bath Light" {
                tunnel: ["MBL/F" "MBL/T"] -> w695
                frame False {
                }
                frame True {
                }
              }
            }
            event "Master Bedroom W.I.C. Light": Value Change {
              n250 = event-data() -> ()  [unwired: 1 in, 1 out]
              n251 = case shown="False" "Master Bedroom W.I.C. Light" {
                tunnel: ["MBWICL/F" "MBWICL/T"] -> w699
                frame False {
                }
                frame True {
                }
              }
            }
            event "Bedroom 2 Light 1": Value Change {
              n252 = event-data() -> ()  [unwired: 1 in, 1 out]
              n253 = case shown="False" "Bedroom 2 Light 1" {
                tunnel: ["B2L1/F" "B2L1/T"] -> w703
                frame False {
                }
                frame True {
                }
              }
            }
            event "Bedroom 2 Light 2": Value Change {
              n254 = event-data() -> ()  [unwired: 1 in, 1 out]
              n255 = case shown="False" "Bedroom 2 Light 2" {
                tunnel: ["B2L2/F" "B2L2/T"] -> w707
                frame False {
                }
                frame True {
                }
              }
            }
            event "Bedroom 2 W.I.C. Light": Value Change {
              n256 = event-data() -> ()  [unwired: 1 in, 1 out]
              n257 = case shown="False" "Bedroom 2 W.I.C. Light" {
                tunnel: ["B2WICL/F" "B2WICL/T"] -> w711
                frame False {
                }
                frame True {
                }
              }
            }
            event "Bedroom 3 Light 1": Value Change {
              n258 = event-data() -> ()  [unwired: 1 in, 1 out]
              n259 = case shown="False" "Bedroom 3 Light 1" {
                tunnel: ["B3L1/F" "B3L1/T"] -> w715
                frame False {
                }
                frame True {
                }
              }
            }
            event "Bedroom 3 Light 2": Value Change {
              n260 = event-data() -> ()  [unwired: 1 in, 1 out]
              n261 = case shown="False" "Bedroom 3 Light 2" {
                tunnel: ["B3L2/F" "B3L2/T"] -> w719
                frame False {
                }
                frame True {
                }
              }
            }
            event "Kitchen Light 1": Value Change {
              n262 = event-data() -> ()  [unwired: 1 in, 1 out]
              n263 = case shown="False" "Kitchen Light 1" {
                tunnel: ["KL1/F" "KL1/T"] -> w723
                frame False {
                }
                frame True {
                }
              }
            }
            event "Kitchen Light 2": Value Change {
              n264 = event-data() -> ()  [unwired: 1 in, 1 out]
              n265 = case shown="False" "Kitchen Light 2" {
                tunnel: ["KL2/F" "KL2/T"] -> w727
                frame False {
                }
                frame True {
                }
              }
            }
            event "T&B Light": Value Change {
              n266 = event-data() -> ()  [unwired: 1 in, 1 out]
              n267 = case shown="False" "T&B Light" {
                tunnel: ["TBL/F" "TBL/T"] -> w731
                frame False {
                }
                frame True {
                }
              }
            }
            event "Lanai Light": Value Change {
              n268 = event-data() -> ()  [unwired: 1 in, 1 out]
              n269 = case shown="False" "Lanai Light" {
                tunnel: ["LL/F" "LL/T"] -> w735
                frame False {
                }
                frame True {
                }
              }
            }
            event "Service Laundry Light 1": Value Change {
              n270 = event-data() -> ()  [unwired: 1 in, 1 out]
              n271 = case shown="False" "Service Laundry Light 1" {
                tunnel: ["SLL1/F" "SLL1/T"] -> w739
                frame False {
                }
                frame True {
                }
              }
            }
            event "Service Laundry Light 2": Value Change {
              n272 = event-data() -> ()  [unwired: 1 in, 1 out]
              n273 = case shown="False" "Service Laundry Light 2" {
                tunnel: ["SLL2/F" "SLL2/T"] -> w743
                frame False {
                }
                frame True {
                }
              }
            }
            event "Garage Light 1": Value Change {
              n274 = event-data() -> ()  [unwired: 1 in, 1 out]
              n275 = case shown="True" "Garage Light 1" {
                tunnel: ["GL1/F" "GL1/T"] -> w747
                frame False {
                }
                frame True {
                }
              }
            }
            event "Garage Light 2": Value Change {
              n276 = event-data() -> ()  [unwired: 1 in, 1 out]
              n277 = case shown="True" "Garage Light 2" {
                tunnel: ["GL2/F" "GL2/T"] -> w751
                frame False {
                }
                frame True {
                }
              }
            }
          }
          n278 = String Length(string=w617) -> (length=w616:i32)
          n279 = Type Cast(x=w616) -> (*(type *) &x=w615:string)  [unwired: 1 in]
          n280 = TCP Write "TCP Write\nCarrying Info\nString Length"(connection ID=w613, data in=w615, error in (no error)=w614) -> (connection ID out=w619:refnum<k5>, error out=w618:errorcluster)  [unwired: 1 in, 1 out]
          n281 = TCP Write "TCP Write\nCarrying\nData"(connection ID=w619, data in=w617, error in (no error)=w618) -> (connection ID out=w611:refnum<k5>, error out=w612:errorcluster)  [unwired: 1 in, 1 out]
        }
        n282 = TCP Open Connection "TCP Open \nConnection"(address="localhost", remote port or service name=u16 51111) -> (connection ID=w223:refnum<k5>, error out=w222:errorcluster)  [unwired: 3 in]
        n283 = while "TV" {
          tunnel: w222 -> [w585]
          tunnel: w223 -> [w584]
          tunnel: [w583] -> w225
          tunnel: [w582] -> w226
          stop <- FALSE stop-if-true
          n284 = event shown="[10] \"Mute\": Value Change" {
            selector: _ -> [_ _ _ _ _ _ _ _ _ _ _ _]
            dyn-events: _ -> [_ _ _ _ _ _ _ _ _ _ _ _]
            timeout: _ -> [_ _ _ _ _ _ _ _ _ _ _ _]
            tunnel: ["ONOF" ("string") "PLAY" ("string") "PAUS" ("string") "STOP" ("string") "FFWD" ("string") "FRWD" ("string") "C1" ("string") "C2" ("string") "C3" ("string") "C4" ("string") w602 w607] -> w588
            event "On/Off": Value Change {
              n285 = event-data() -> ()  [unwired: 1 in, 1 out]
            }
            event "Play": Value Change {
              n286 = event-data() -> ()  [unwired: 1 in, 1 out]
            }
            event "Pause": Value Change {
              n287 = event-data() -> ()  [unwired: 1 in, 1 out]
            }
            event "Stop": Value Change {
              n288 = event-data() -> ()  [unwired: 1 in, 1 out]
            }
            event "Fast Forward": Value Change {
              n289 = event-data() -> ()  [unwired: 1 in, 1 out]
            }
            event "Fast Reverse": Value Change {
              n290 = event-data() -> ()  [unwired: 1 in, 1 out]
            }
            event "Channel 1": Value Change {
              n291 = event-data() -> ()  [unwired: 1 in, 1 out]
            }
            event "Channel 2": Value Change {
              n292 = event-data() -> ()  [unwired: 1 in, 1 out]
            }
            event "Channel 3": Value Change {
              n293 = event-data() -> ()  [unwired: 1 in, 1 out]
            }
            event "Channel 4": Value Change {
              n294 = event-data() -> ()  [unwired: 1 in, 1 out]
            }
            event "Mute": Value Change {
              n295 = event-data() -> ()  [unwired: 1 in, 1 out]
              n296 = Type Cast(x="Mute") -> (*(type *) &x=w604:string)  [unwired: 1 in]
              n297 = Concatenate Strings "Concatenate Strings"("MUTE" ("string"), w604) -> (w602:string)
            }
            event "Volume": Value Change {
              n298 = event-data() -> ()  [unwired: 1 in, 1 out]
              n299 = Type Cast(x="Volume") -> (*(type *) &x=w609:string)  [unwired: 1 in]
              n300 = Concatenate Strings "Concatenate Strings"("VOLM" ("string"), w609) -> (w607:string)
            }
          }
          n301 = String Length(string=w588) -> (length=w589:i32)
          n302 = Type Cast(x=w589) -> (*(type *) &x=w587:string)  [unwired: 1 in]
          n303 = TCP Write "TCP Write\nCarrying Info\nString Length"(connection ID=w584, data in=w587, error in (no error)=w585) -> (connection ID out=w590:refnum<k5>, error out=w591:errorcluster)  [unwired: 1 in, 1 out]
          n304 = TCP Write "TCP Write\nCarrying\nData"(connection ID=w590, data in=w588, error in (no error)=w591) -> (connection ID out=w582:refnum<k5>, error out=w583:errorcluster)  [unwired: 1 in, 1 out]
        }
        n305 = TCP Close Connection "TCP Close \nConnection"(connection ID=w226, error in (no error)=w225) -> (error out=w224:errorcluster)  [unwired: 1 in, 1 out]
        n306 = call <vilib>:"Clear Errors.vi"("error in (no error)"=w224) -> ()  [unwired: 5 in, 2 out]
        n307 = TCP Close Connection "TCP Close \nConnection"(connection ID=w227, error in (no error)=w228) -> (error out=w229:errorcluster)  [unwired: 1 in, 1 out]
        n308 = call <vilib>:"Clear Errors.vi"("error in (no error)"=w229) -> ()  [unwired: 5 in, 2 out]
        n309 = TCP Open Connection "TCP Open \nConnection"(address="localhost", remote port or service name=u16 51112, timeout ms (60000)=60000) -> (connection ID=w215:refnum<k5>, error out=w219:errorcluster)  [unwired: 2 in]
        n310 = TCP Open Connection "TCP Open \nConnection"(address="localhost", remote port or service name=u16 51113) -> (connection ID=w208:refnum<k5>, error out=w207:errorcluster)  [unwired: 3 in]
        n311 = while "Main Control" {
          tunnel: w215 -> [w489]
          tunnel: [w487] -> w216
          tunnel: [w486] -> w217
          tunnel: w219 -> [w484]
          stop <- FALSE stop-if-true
          n312 = event shown="[1] \"Clock\": Value Change" {
            selector: _ -> [_ _ _ _ _ _ _ _]
            dyn-events: _ -> [_ _ _ _ _ _ _ _]
            timeout: _ -> [_ _ _ _ _ _ _ _]
            tunnel: [w503 w520 w526 w556 w561 w568 w572 w576] -> w481
            event "Temperature(°C)": Value Change {
              n313 = event-data() -> ()  [unwired: 1 in, 1 out]
              n314 = local read "Temperature(°C)"() -> (w499:dbl)
              n315 = local read "Temperature(°C)"() -> (w492:dbl)
              n316 = Greater?(x=w499, y=30.0) -> (0:w497:bool)
              n317 = Greater Or Equal?(x=w492, y=50.0) -> (x >= y?=w491:bool)
              n318 = case shown="True" w491 {
                frame False {
                }
                frame True {
                  w508 = 0.0 ("Bedroom 3 Curtain 1")
                  w509 = FALSE ("Main Door")
                  n319 = local write "Bedroom 2 Door"(w509) -> ()
                  n320 = local write "Bedroom 3 Door"(w509) -> ()
                  n321 = local write "Master Bedroom Door"(w509) -> ()
                  n322 = local write "Master Bath Door"(w509) -> ()
                  n323 = local write "Lanai Door"(w509) -> ()
                  n324 = local write "T&B Door"(w509) -> ()
                  n325 = local write "Service/Laundry Door"(w509) -> ()
                  n326 = local write "Main Door"(w509) -> ()
                  n327 = local write "Master Curtain"(FALSE ("Master Curtain")) -> ()
                  n328 = local write "Master Door"(TRUE ("Master Door")) -> ()
                  n329 = local write "Kitchen Curtain 2"(w508) -> ()
                  n330 = local write "Kitchen Curtain 1"(w508) -> ()
                  n331 = local write "Bedroom 3 Curtain 2"(w508) -> ()
                  n332 = local write "Bedroom 3 Curtain 1"(w508) -> ()
                  n333 = local write "Bedroom 2 Curtain 2"(w508) -> ()
                  n334 = local write "Bedroom 2 Curtain 1"(w508) -> ()
                  n335 = local write "Master Bedroom Curtain"(w508) -> ()
                  n336 = local write "Living Area Curtain"(w508) -> ()
                }
              }
              n337 = case shown="True" w497 {
                frame False {
                }
                frame True {
                  w511 = TRUE ("Bedroom 3 AirCon")
                  n338 = local write "Master Bedroom AirCon"(w511) -> ()
                  n339 = local write "Bedroom 3 AirCon"(w511) -> ()
                  n340 = local write "Bedroom 2 AirCon"(w511) -> ()
                  n341 = local write "Living Area AirCon"(w511) -> ()
                }
              }
              n342 = local read "Temperature(°C)"() -> (w502:dbl)
              n343 = local read "Temperature(°C)"() -> (w494:dbl)
              n344 = Format Into String "Format Into String"(format string="%02d", w502) -> (resulting string=w501:string)  [unwired: 2 in, 1 out]
              n345 = Concatenate Strings "Concatenate Strings"("TEMPE" ("string"), w501) -> (w503:string)
              n346 = Less?(x=w494, y=10.0) -> (x < y?=w496:bool)
              n347 = case shown="True" w496 {
                frame False {
                }
                frame True {
                  w510 = FALSE ("Bedroom 3 AirCon")
                  n348 = local write "Master Bedroom AirCon"(w510) -> ()
                  n349 = local write "Bedroom 3 AirCon"(w510) -> ()
                  n350 = local write "Bedroom 2 AirCon"(w510) -> ()
                  n351 = local write "Living Area AirCon"(w510) -> ()
                }
              }
              "Temperature(°C)" <- "Temperature(°C)"
            }
            event "Clock": Value Change {
              n352 = event-data() -> ()  [unwired: 1 in, 1 out]
              n353 = Seconds To Date/Time(time stamp (now)="Clock") -> (date time rec=w517:T4)  [unwired: 1 in]
              n354 = Unbundle By Name "Unbundle By Name"(w517) -> ("hour"=w516:i32)
              n355 = In Range and Coerce(upper limit=19, x=w516, lower limit=7) -> (In Range?=w512:bool)  [unwired: 1 out]
              n356 = Type Cast(x=w512) -> (*(type *) &x=w513:string)  [unwired: 1 in]
              n357 = Concatenate Strings "Concatenate Strings"("CLOCK" ("string"), w513) -> (w520:string)
              n358 = case shown="True" w512 {
                frame False {
                  w522 = 100.0 ("Bedroom 3 Curtain 1")
                  n359 = local write "Kitchen Curtain 2"(w522) -> ()
                  n360 = local write "Kitchen Curtain 1"(w522) -> ()
                  n361 = local write "Bedroom 3 Curtain 2"(w522) -> ()
                  n362 = local write "Bedroom 3 Curtain 1"(w522) -> ()
                  n363 = local write "Bedroom 2 Curtain 2"(w522) -> ()
                  n364 = local write "Bedroom 2 Curtain 1"(w522) -> ()
                  n365 = local write "Master Bedroom Curtain"(w522) -> ()
                  n366 = local write "Living Area Curtain"(w522) -> ()
                  n367 = local write "Master Curtain"(TRUE ("Master Curtain")) -> ()
                }
                frame True {
                  w524 = 0.0 ("Bedroom 3 Curtain 1")
                  n368 = local write "Master Curtain"(FALSE ("Master Curtain")) -> ()
                  n369 = local write "Kitchen Curtain 2"(w524) -> ()
                  n370 = local write "Kitchen Curtain 1"(w524) -> ()
                  n371 = local write "Bedroom 3 Curtain 2"(w524) -> ()
                  n372 = local write "Bedroom 3 Curtain 1"(w524) -> ()
                  n373 = local write "Bedroom 2 Curtain 2"(w524) -> ()
                  n374 = local write "Bedroom 2 Curtain 1"(w524) -> ()
                  n375 = local write "Master Bedroom Curtain"(w524) -> ()
                  n376 = local write "Living Area Curtain"(w524) -> ()
                }
              }
            }
            event "Master Light": Value Change {
              n377 = event-data() -> ()  [unwired: 1 in, 1 out]
              n378 = case shown="False" "Master Light" {
                frame False {
                  w529 = T5."Enabled" ("Disabled")
                  n379 = property on="Porch Light" class="Bool (strict)"("DisabledEnum"=w529) -> ()  [unwired: 2 in, 2 out]
                  n380 = property on="Living Area Light 1" class="Bool (strict)"("DisabledEnum"=w529) -> ()  [unwired: 2 in, 2 out]
                  n381 = property on="Living Area Light 2" class="Bool (strict)"("DisabledEnum"=w529) -> ()  [unwired: 2 in, 2 out]
                  n382 = property on="Dining Area Light 1" class="Bool (strict)"("DisabledEnum"=w529) -> ()  [unwired: 2 in, 2 out]
                  n383 = property on="Dining Area Light 2" class="Bool (strict)"("DisabledEnum"=w529) -> ()  [unwired: 2 in, 2 out]
                  n384 = property on="Master Bedroom Light 1" class="Bool (strict)"("DisabledEnum"=w529) -> ()  [unwired: 2 in, 2 out]
                  n385 = property on="Master Bedroom Light 2" class="Bool (strict)"("DisabledEnum"=w529) -> ()  [unwired: 2 in, 2 out]
                  n386 = property on="Master Bath Light" class="Bool (strict)"("DisabledEnum"=w529) -> ()  [unwired: 2 in, 2 out]
                  n387 = property on="Master Bedroom W.I.C. Light" class="Bool (strict)"("DisabledEnum"=w529) -> ()  [unwired: 2 in, 2 out]
                  n388 = property on="Bedroom 2 Light 1" class="Bool (strict)"("DisabledEnum"=w529) -> ()  [unwired: 2 in, 2 out]
                  n389 = property on="Bedroom 2 Light 2" class="Bool (strict)"("DisabledEnum"=w529) -> ()  [unwired: 2 in, 2 out]
                  n390 = property on="Bedroom 2 W.I.C. Light" class="Bool (strict)"("DisabledEnum"=w529) -> ()  [unwired: 2 in, 2 out]
                  n391 = property on="Bedroom 3 Light 1" class="Bool (strict)"("DisabledEnum"=w529) -> ()  [unwired: 2 in, 2 out]
                  n392 = property on="Bedroom 3 Light 2" class="Bool (strict)"("DisabledEnum"=w529) -> ()  [unwired: 2 in, 2 out]
                  n393 = property on="Kitchen Light 1" class="Bool (strict)"("DisabledEnum"=w529) -> ()  [unwired: 2 in, 2 out]
                  n394 = property on="Kitchen Light 2" class="Bool (strict)"("DisabledEnum"=w529) -> ()  [unwired: 2 in, 2 out]
                  n395 = property on="T&B Light" class="Bool (strict)"("DisabledEnum"=w529) -> ()  [unwired: 2 in, 2 out]
                  n396 = property on="Lanai Light" class="Bool (strict)"("DisabledEnum"=w529) -> ()  [unwired: 2 in, 2 out]
                  n397 = property on="Service Laundry Light 1" class="Bool (strict)"("DisabledEnum"=w529) -> ()  [unwired: 2 in, 2 out]
                  n398 = property on="Service Laundry Light 2" class="Bool (strict)"("DisabledEnum"=w529) -> ()  [unwired: 2 in, 2 out]
                  n399 = property on="Garage Light 2" class="Bool (strict)"("DisabledEnum"=w529) -> ()  [unwired: 2 in, 2 out]
                  n400 = property on="Garage Light 1" class="Bool (strict)"("DisabledEnum"=w529) -> ()  [unwired: 2 in, 2 out]
                }
                frame True {
                  n401 = flat-sequence {
                    frame #0 {
                      n402 = local write "Porch Light"(FALSE ("Porch Light")) -> ()
                      n403 = local write "Living Area Light 1"(FALSE ("Living Area Light 1")) -> ()
                      n404 = local write "Living Area Light 2"(FALSE ("Living Area Light 2")) -> ()
                      n405 = local write "Dining Area Light 1"(FALSE ("Dining Area Light 1")) -> ()
                      n406 = local write "Dining Area Light 2"(FALSE ("Dining Area Light 2")) -> ()
                      n407 = local write "Master Bedroom Light 1"(FALSE ("Master Bedroom Light 1")) -> ()
                      n408 = local write "Master Bedroom Light 2"(FALSE ("Master Bedroom Light 2")) -> ()
                      n409 = local write "Master Bath Light"(FALSE ("Master Bath Light")) -> ()
                      n410 = local write "Master Bedroom W.I.C. Light"(FALSE ("Master Bedroom W.I.C. Light")) -> ()
                      n411 = local write "Bedroom 2 Light 1"(FALSE ("Bedroom 2 Light 1")) -> ()
                      n412 = local write "Bedroom 2 Light 2"(FALSE ("Bedroom 2 Light 2")) -> ()
                      n413 = local write "Bedroom 2 W.I.C. Light"(FALSE ("Bedroom 2 W.I.C. Light")) -> ()
                      n414 = local write "Bedroom 3 Light 1"(FALSE ("Bedroom 3 Light 1")) -> ()
                      n415 = local write "Bedroom 3 Light 2"(FALSE ("Bedroom 3 Light 2")) -> ()
                      n416 = local write "Kitchen Light 1"(FALSE ("Kitchen Light 1")) -> ()
                      n417 = local write "Kitchen Light 2"(FALSE ("Kitchen Light 2")) -> ()
                      n418 = local write "T&B Light"(FALSE ("T&B Light")) -> ()
                      n419 = local write "Lanai Light"(FALSE ("Lanai Light")) -> ()
                      n420 = local write "Service Laundry Light 1"(FALSE ("Service Laundry Light 1")) -> ()
                      n421 = local write "Service Laundry Light 2"(FALSE ("Service Laundry Light 2")) -> ()
                      n422 = local write "Garage Light 1"(FALSE ("Garage Light 1")) -> ()
                      n423 = local write "Garage Light 2"(FALSE ("Garage Light 2")) -> ()
                    }
                    frame #1 {
                      w552 = T5."Disabled" ("Disabled")
                      n424 = property on="Porch Light" class="Bool (strict)"("DisabledEnum"=w552) -> ()  [unwired: 2 in, 2 out]
                      n425 = property on="Living Area Light 1" class="Bool (strict)"("DisabledEnum"=w552) -> ()  [unwired: 2 in, 2 out]
                      n426 = property on="Living Area Light 2" class="Bool (strict)"("DisabledEnum"=w552) -> ()  [unwired: 2 in, 2 out]
                      n427 = property on="Dining Area Light 1" class="Bool (strict)"("DisabledEnum"=w552) -> ()  [unwired: 2 in, 2 out]
                      n428 = property on="Dining Area Light 2" class="Bool (strict)"("DisabledEnum"=w552) -> ()  [unwired: 2 in, 2 out]
                      n429 = property on="Master Bedroom Light 1" class="Bool (strict)"("DisabledEnum"=w552) -> ()  [unwired: 2 in, 2 out]
                      n430 = property on="Master Bedroom Light 2" class="Bool (strict)"("DisabledEnum"=w552) -> ()  [unwired: 2 in, 2 out]
                      n431 = property on="Master Bath Light" class="Bool (strict)"("DisabledEnum"=w552) -> ()  [unwired: 2 in, 2 out]
                      n432 = property on="Master Bedroom W.I.C. Light" class="Bool (strict)"("DisabledEnum"=w552) -> ()  [unwired: 2 in, 2 out]
                      n433 = property on="Bedroom 2 Light 1" class="Bool (strict)"("DisabledEnum"=w552) -> ()  [unwired: 2 in, 2 out]
                      n434 = property on="Bedroom 2 Light 2" class="Bool (strict)"("DisabledEnum"=w552) -> ()  [unwired: 2 in, 2 out]
                      n435 = property on="Bedroom 2 W.I.C. Light" class="Bool (strict)"("DisabledEnum"=w552) -> ()  [unwired: 2 in, 2 out]
                      n436 = property on="Bedroom 3 Light 1" class="Bool (strict)"("DisabledEnum"=w552) -> ()  [unwired: 2 in, 2 out]
                      n437 = property on="Bedroom 3 Light 2" class="Bool (strict)"("DisabledEnum"=w552) -> ()  [unwired: 2 in, 2 out]
                      n438 = property on="Kitchen Light 1" class="Bool (strict)"("DisabledEnum"=w552) -> ()  [unwired: 2 in, 2 out]
                      n439 = property on="Kitchen Light 2" class="Bool (strict)"("DisabledEnum"=w552) -> ()  [unwired: 2 in, 2 out]
                      n440 = property on="T&B Light" class="Bool (strict)"("DisabledEnum"=w552) -> ()  [unwired: 2 in, 2 out]
                      n441 = property on="Lanai Light" class="Bool (strict)"("DisabledEnum"=w552) -> ()  [unwired: 2 in, 2 out]
                      n442 = property on="Service Laundry Light 1" class="Bool (strict)"("DisabledEnum"=w552) -> ()  [unwired: 2 in, 2 out]
                      n443 = property on="Service Laundry Light 2" class="Bool (strict)"("DisabledEnum"=w552) -> ()  [unwired: 2 in, 2 out]
                      n444 = property on="Garage Light 2" class="Bool (strict)"("DisabledEnum"=w552) -> ()  [unwired: 2 in, 2 out]
                      n445 = property on="Garage Light 1" class="Bool (strict)"("DisabledEnum"=w552) -> ()  [unwired: 2 in, 2 out]
                    }
                  }
                }
              }
              n446 = Type Cast(x="Master Light") -> (*(type *) &x=w528:string)  [unwired: 1 in]
              n447 = Concatenate Strings "Concatenate Strings"("MAINL" ("string"), w528) -> (w526:string)
            }
            event "Master Door": Value Change {
              n448 = event-data() -> ()  [unwired: 1 in, 1 out]
              n449 = case shown="True" "Master Door" {
                frame False {
                  w557 = T5."Enabled" ("Disabled")
                  n450 = property on="Main Door" class="Bool (strict)"("DisabledEnum"=w557) -> ()  [unwired: 2 in, 2 out]
                  n451 = property on="Bedroom 2 Door" class="Bool (strict)"("DisabledEnum"=w557) -> ()  [unwired: 2 in, 2 out]
                  n452 = property on="Bedroom 3 Door" class="Bool (strict)"("DisabledEnum"=w557) -> ()  [unwired: 2 in, 2 out]
                  n453 = property on="Master Bedroom Door" class="Bool (strict)"("DisabledEnum"=w557) -> ()  [unwired: 2 in, 2 out]
                  n454 = property on="Master Bath Door" class="Bool (strict)"("DisabledEnum"=w557) -> ()  [unwired: 2 in, 2 out]
                  n455 = property on="Lanai Door" class="Bool (strict)"("DisabledEnum"=w557) -> ()  [unwired: 2 in, 2 out]
                  n456 = property on="T&B Door" class="Bool (strict)"("DisabledEnum"=w557) -> ()  [unwired: 2 in, 2 out]
                  n457 = property on="Service/Laundry Door" class="Bool (strict)"("DisabledEnum"=w557) -> ()  [unwired: 2 in, 2 out]
                }
                frame True {
                  n458 = flat-sequence {
                    frame #0 {
                      w558 = FALSE ("Main Door")
                      n459 = local write "Bedroom 2 Door"(w558) -> ()
                      n460 = local write "Bedroom 3 Door"(w558) -> ()
                      n461 = local write "Master Bedroom Door"(w558) -> ()
                      n462 = local write "Master Bath Door"(w558) -> ()
                      n463 = local write "Lanai Door"(w558) -> ()
                      n464 = local write "T&B Door"(w558) -> ()
                      n465 = local write "Service/Laundry Door"(w558) -> ()
                      n466 = local write "Main Door"(w558) -> ()
                    }
                    frame #1 {
                      w559 = T5."Disabled" ("Disabled")
                      n467 = property on="Main Door" class="Bool (strict)"("DisabledEnum"=w559) -> ()  [unwired: 2 in, 2 out]
                      n468 = property on="Bedroom 2 Door" class="Bool (strict)"("DisabledEnum"=w559) -> ()  [unwired: 2 in, 2 out]
                      n469 = property on="Bedroom 3 Door" class="Bool (strict)"("DisabledEnum"=w559) -> ()  [unwired: 2 in, 2 out]
                      n470 = property on="Master Bedroom Door" class="Bool (strict)"("DisabledEnum"=w559) -> ()  [unwired: 2 in, 2 out]
                      n471 = property on="Master Bath Door" class="Bool (strict)"("DisabledEnum"=w559) -> ()  [unwired: 2 in, 2 out]
                      n472 = property on="Lanai Door" class="Bool (strict)"("DisabledEnum"=w559) -> ()  [unwired: 2 in, 2 out]
                      n473 = property on="T&B Door" class="Bool (strict)"("DisabledEnum"=w559) -> ()  [unwired: 2 in, 2 out]
                      n474 = property on="Service/Laundry Door" class="Bool (strict)"("DisabledEnum"=w559) -> ()  [unwired: 2 in, 2 out]
                    }
                  }
                }
              }
              n475 = Type Cast(x="Master Door") -> (*(type *) &x=w554:string)  [unwired: 1 in]
              n476 = Concatenate Strings "Concatenate Strings"("MAIND" ("string"), w554) -> (w556:string)
            }
            event "Master Curtain": Value Change {
              n477 = event-data() -> ()  [unwired: 1 in, 1 out]
              n478 = case shown="True" "Master Curtain" {
                frame False {
                  w564 = T5."Enabled" ("Disabled")
                  n479 = property on="Master Bedroom Curtain" class="Slide (strict)"("DisabledEnum"=w564) -> ()  [unwired: 2 in, 2 out]
                  n480 = property on="Living Area Curtain" class="Slide (strict)"("DisabledEnum"=w564) -> ()  [unwired: 2 in, 2 out]
                  n481 = property on="Kitchen Curtain 2" class="Slide (strict)"("DisabledEnum"=w564) -> ()  [unwired: 2 in, 2 out]
                  n482 = property on="Kitchen Curtain 1" class="Slide (strict)"("DisabledEnum"=w564) -> ()  [unwired: 2 in, 2 out]
                  n483 = property on="Bedroom 3 Curtain 2" class="Slide (strict)"("DisabledEnum"=w564) -> ()  [unwired: 2 in, 2 out]
                  n484 = property on="Bedroom 3 Curtain 1" class="Slide (strict)"("DisabledEnum"=w564) -> ()  [unwired: 2 in, 2 out]
                  n485 = property on="Bedroom 2 Curtain 2" class="Slide (strict)"("DisabledEnum"=w564) -> ()  [unwired: 2 in, 2 out]
                  n486 = property on="Bedroom 2 Curtain 1" class="Slide (strict)"("DisabledEnum"=w564) -> ()  [unwired: 2 in, 2 out]
                }
                frame True {
                  n487 = flat-sequence {
                    frame #0 {
                      w565 = 0.0 ("Bedroom 3 Curtain 1")
                      n488 = local write "Kitchen Curtain 2"(w565) -> ()
                      n489 = local write "Kitchen Curtain 1"(w565) -> ()
                      n490 = local write "Bedroom 3 Curtain 2"(w565) -> ()
                      n491 = local write "Bedroom 3 Curtain 1"(w565) -> ()
                      n492 = local write "Bedroom 2 Curtain 2"(w565) -> ()
                      n493 = local write "Bedroom 2 Curtain 1"(w565) -> ()
                      n494 = local write "Master Bedroom Curtain"(w565) -> ()
                      n495 = local write "Living Area Curtain"(w565) -> ()
                    }
                    frame #1 {
                      w566 = T5."Disabled" ("Disabled")
                      n496 = property on="Master Bedroom Curtain" class="Slide (strict)"("DisabledEnum"=w566) -> ()  [unwired: 2 in, 2 out]
                      n497 = property on="Living Area Curtain" class="Slide (strict)"("DisabledEnum"=w566) -> ()  [unwired: 2 in, 2 out]
                      n498 = property on="Kitchen Curtain 2" class="Slide (strict)"("DisabledEnum"=w566) -> ()  [unwired: 2 in, 2 out]
                      n499 = property on="Kitchen Curtain 1" class="Slide (strict)"("DisabledEnum"=w566) -> ()  [unwired: 2 in, 2 out]
                      n500 = property on="Bedroom 3 Curtain 2" class="Slide (strict)"("DisabledEnum"=w566) -> ()  [unwired: 2 in, 2 out]
                      n501 = property on="Bedroom 3 Curtain 1" class="Slide (strict)"("DisabledEnum"=w566) -> ()  [unwired: 2 in, 2 out]
                      n502 = property on="Bedroom 2 Curtain 2" class="Slide (strict)"("DisabledEnum"=w566) -> ()  [unwired: 2 in, 2 out]
                      n503 = property on="Bedroom 2 Curtain 1" class="Slide (strict)"("DisabledEnum"=w566) -> ()  [unwired: 2 in, 2 out]
                    }
                  }
                }
              }
              n504 = Type Cast(x="Master Curtain") -> (*(type *) &x=w563:string)  [unwired: 1 in]
              n505 = Concatenate Strings "Concatenate Strings"("MAINW" ("string"), w563) -> (w561:string)
            }
            event "Holiday Mode": Value Change {
              n506 = event-data() -> ()  [unwired: 1 in, 1 out]
              n507 = Type Cast(x="Holiday Mode") -> (*(type *) &x=w570:string)  [unwired: 1 in]
              n508 = Concatenate Strings "Concatenate Strings"("HLDMD" ("string"), w570) -> (w568:string)
            }
            event "Door Automatically Open": Value Change {
              n509 = event-data() -> ()  [unwired: 1 in, 1 out]
              n510 = Type Cast(x="Door Automatically Open") -> (*(type *) &x=w574:string)  [unwired: 1 in]
              n511 = Concatenate Strings "Concatenate Strings"("DRAOP" ("string"), w574) -> (w572:string)
            }
            event "Alarm System": Value Change {
              n512 = event-data() -> ()  [unwired: 1 in, 1 out]
              n513 = case shown="False" "Alarm System" {
                frame False {
                  w579 = T5."Enabled" ("Disabled")
                  n514 = property on="Service/Laundry Door" class="Bool (strict)"("DisabledEnum"=w579) -> ()  [unwired: 2 in, 2 out]
                  n515 = property on="Main Door" class="Bool (strict)"("DisabledEnum"=w579) -> ()  [unwired: 2 in, 2 out]
                  n516 = property on="Master Door" class="Bool (strict)"("DisabledEnum"=w579) -> ()  [unwired: 2 in, 2 out]
                  n517 = property on="Lanai Door" class="Bool (strict)"("DisabledEnum"=w579) -> ()  [unwired: 2 in, 2 out]
                }
                frame True {
                  n518 = flat-sequence {
                    frame #0 {
                      w580 = FALSE ("Main Door")
                      n519 = local write "Master Door"(w580) -> ()
                      n520 = local write "Main Door"(w580) -> ()
                      n521 = local write "Lanai Door"(w580) -> ()
                      n522 = local write "Service/Laundry Door"(w580) -> ()
                    }
                    frame #1 {
                      w581 = T5."Disabled" ("Disabled")
                      n523 = property on="Service/Laundry Door" class="Bool (strict)"("DisabledEnum"=w581) -> ()  [unwired: 2 in, 2 out]
                      n524 = property on="Main Door" class="Bool (strict)"("DisabledEnum"=w581) -> ()  [unwired: 2 in, 2 out]
                      n525 = property on="Lanai Door" class="Bool (strict)"("DisabledEnum"=w581) -> ()  [unwired: 2 in, 2 out]
                      n526 = property on="Master Door" class="Bool (strict)"("DisabledEnum"=w581) -> ()  [unwired: 2 in, 2 out]
                    }
                  }
                }
              }
              n527 = Type Cast(x="Alarm System") -> (*(type *) &x=w578:string)  [unwired: 1 in]
              n528 = Concatenate Strings "Concatenate Strings"("ALARM" ("string"), w578) -> (w576:string)
            }
          }
          n529 = String Length(string=w481) -> (length=w483:i32)
          n530 = Type Cast(x=w483) -> (*(type *) &x=w482:string)  [unwired: 1 in]
          n531 = TCP Write "TCP Write\nCarrying Info\nString Length"(connection ID=w489, data in=w482, error in (no error)=w484) -> (connection ID out=w488:refnum<k5>, error out=w485:errorcluster)  [unwired: 1 in, 1 out]
          n532 = TCP Write "TCP Write\nCarrying\nData"(connection ID=w488, data in=w481, error in (no error)=w485) -> (connection ID out=w487:refnum<k5>, error out=w486:errorcluster)  [unwired: 1 in, 1 out]
        }
        n533 = while "Door" {
          tunnel: w207 -> [w443]
          tunnel: w208 -> [w442]
          tunnel: [w441] -> w210
          tunnel: [w440] -> w211
          stop <- FALSE stop-if-true
          n534 = event shown="[2] \"Bedroom 3 Door\": Value Change" {
            selector: _ -> [_ _ _ _ _ _ _ _]
            dyn-events: _ -> [_ _ _ _ _ _ _ _]
            timeout: _ -> [_ _ _ _ _ _ _ _]
            tunnel: [w452 w455 w459 w463 w467 w471 w475 w479] -> w439
            event "Main Door": Value Change {
              n535 = event-data() -> ()  [unwired: 1 in, 1 out]
              n536 = Type Cast(x="Main Door") -> (*(type *) &x=w450:string)  [unwired: 1 in]
              n537 = Concatenate Strings "Concatenate Strings"("MD" ("string"), w450) -> (w452:string)
            }
            event "Bedroom 2 Door": Value Change {
              n538 = event-data() -> ()  [unwired: 1 in, 1 out]
              n539 = Type Cast(x="Bedroom 2 Door") -> (*(type *) &x=w456:string)  [unwired: 1 in]
              n540 = Concatenate Strings "Concatenate Strings"("B2" ("string"), w456) -> (w455:string)
            }
            event "Bedroom 3 Door": Value Change {
              n541 = event-data() -> ()  [unwired: 1 in, 1 out]
              n542 = Type Cast(x="Bedroom 3 Door") -> (*(type *) &x=w460:string)  [unwired: 1 in]
              n543 = Concatenate Strings "Concatenate Strings"("B3" ("string"), w460) -> (w459:string)
            }
            event "Master Bedroom Door": Value Change {
              n544 = event-data() -> ()  [unwired: 1 in, 1 out]
              n545 = Type Cast(x="Master Bedroom Door") -> (*(type *) &x=w464:string)  [unwired: 1 in]
              n546 = Concatenate Strings "Concatenate Strings"("B1" ("string"), w464) -> (w463:string)
            }
            event "Master Bath Door": Value Change {
              n547 = event-data() -> ()  [unwired: 1 in, 1 out]
              n548 = Type Cast(x="Master Bath Door") -> (*(type *) &x=w468:string)  [unwired: 1 in]
              n549 = Concatenate Strings "Concatenate Strings"("MB" ("string"), w468) -> (w467:string)
            }
            event "Lanai Door": Value Change {
              n550 = event-data() -> ()  [unwired: 1 in, 1 out]
              n551 = Type Cast(x="Lanai Door") -> (*(type *) &x=w472:string)  [unwired: 1 in]
              n552 = Concatenate Strings "Concatenate Strings"("LA" ("string"), w472) -> (w471:string)
            }
            event "T&B Door": Value Change {
              n553 = event-data() -> ()  [unwired: 1 in, 1 out]
              n554 = Type Cast(x="T&B Door") -> (*(type *) &x=w476:string)  [unwired: 1 in]
              n555 = Concatenate Strings "Concatenate Strings"("TB" ("string"), w476) -> (w475:string)
            }
            event "Service/Laundry Door": Value Change {
              n556 = event-data() -> ()  [unwired: 1 in, 1 out]
              n557 = Type Cast(x="Service/Laundry Door") -> (*(type *) &x=w480:string)  [unwired: 1 in]
              n558 = Concatenate Strings "Concatenate Strings"("SL" ("string"), w480) -> (w479:string)
            }
          }
          n559 = String Length(string=w439) -> (length=w446:i32)
          n560 = Type Cast(x=w446) -> (*(type *) &x=w445:string)  [unwired: 1 in]
          n561 = TCP Write "TCP Write\nCarrying Info\nString Length"(connection ID=w442, data in=w445, error in (no error)=w443) -> (connection ID out=w447:refnum<k5>, error out=w448:errorcluster)  [unwired: 1 in, 1 out]
          n562 = TCP Write "TCP Write\nCarrying\nData"(connection ID=w447, data in=w439, error in (no error)=w448) -> (connection ID out=w440:refnum<k5>, error out=w441:errorcluster)  [unwired: 1 in, 1 out]
        }
        n563 = TCP Close Connection "TCP Close \nConnection"(connection ID=w211, error in (no error)=w210) -> (error out=w209:errorcluster)  [unwired: 1 in, 1 out]
        n564 = call <vilib>:"Clear Errors.vi"("error in (no error)"=w209) -> ()  [unwired: 5 in, 2 out]
        n565 = TCP Open Connection "TCP Open \nConnection"(address="localhost", remote port or service name=u16 51114) -> (connection ID=w201:refnum<k5>, error out=w202:errorcluster)  [unwired: 3 in]
        n566 = while "Curtain" {
          tunnel: w202 -> [w385]
          tunnel: w201 -> [w384]
          tunnel: [w383] -> w199
          tunnel: [w382] -> w198
          stop <- FALSE stop-if-true
          n567 = event shown="[0] \"Living Area Curtain\": Value Change" {
            selector: _ -> [_ _ _ _ _ _ _ _]
            dyn-events: _ -> [_ _ _ _ _ _ _ _]
            timeout: _ -> [_ _ _ _ _ _ _ _]
            tunnel: [w394 w400 w406 w412 w418 w424 w430 w436] -> w381
            event "Living Area Curtain": Value Change {
              n568 = event-data() -> ()  [unwired: 1 in, 1 out]
              n569 = Format Into String "Format Into String"(format string="%03d", "Living Area Curtain") -> (resulting string=w391:string)  [unwired: 2 in, 1 out]
              n570 = Type Cast(x=w391) -> (*(type *) &x=w395:string)  [unwired: 1 in]
              n571 = Concatenate Strings "Concatenate Strings"("00" ("string"), w395) -> (w394:string)
            }
            event "Master Bedroom Curtain": Value Change {
              n572 = event-data() -> ()  [unwired: 1 in, 1 out]
              n573 = Format Into String "Format Into String"(format string="%03d", "Master Bedroom Curtain") -> (resulting string=w398:string)  [unwired: 2 in, 1 out]
              n574 = Type Cast(x=w398) -> (*(type *) &x=w401:string)  [unwired: 1 in]
              n575 = Concatenate Strings "Concatenate Strings"("01" ("string"), w401) -> (w400:string)
            }
            event "Bedroom 2 Curtain 1": Value Change {
              n576 = event-data() -> ()  [unwired: 1 in, 1 out]
              n577 = Format Into String "Format Into String"(format string="%03d", "Bedroom 2 Curtain 1") -> (resulting string=w404:string)  [unwired: 2 in, 1 out]
              n578 = Type Cast(x=w404) -> (*(type *) &x=w407:string)  [unwired: 1 in]
              n579 = Concatenate Strings "Concatenate Strings"("02" ("string"), w407) -> (w406:string)
            }
            event "Bedroom 2 Curtain 2": Value Change {
              n580 = event-data() -> ()  [unwired: 1 in, 1 out]
              n581 = Format Into String "Format Into String"(format string="%03d", "Bedroom 2 Curtain 2") -> (resulting string=w410:string)  [unwired: 2 in, 1 out]
              n582 = Type Cast(x=w410) -> (*(type *) &x=w413:string)  [unwired: 1 in]
              n583 = Concatenate Strings "Concatenate Strings"("03" ("string"), w413) -> (w412:string)
            }
            event "Bedroom 3 Curtain 1": Value Change {
              n584 = event-data() -> ()  [unwired: 1 in, 1 out]
              n585 = Format Into String "Format Into String"(format string="%03d", "Bedroom 3 Curtain 1") -> (resulting string=w416:string)  [unwired: 2 in, 1 out]
              n586 = Type Cast(x=w416) -> (*(type *) &x=w419:string)  [unwired: 1 in]
              n587 = Concatenate Strings "Concatenate Strings"("04" ("string"), w419) -> (w418:string)
            }
            event "Bedroom 3 Curtain 2": Value Change {
              n588 = event-data() -> ()  [unwired: 1 in, 1 out]
              n589 = Format Into String "Format Into String"(format string="%03d", "Bedroom 3 Curtain 2") -> (resulting string=w422:string)  [unwired: 2 in, 1 out]
              n590 = Type Cast(x=w422) -> (*(type *) &x=w425:string)  [unwired: 1 in]
              n591 = Concatenate Strings "Concatenate Strings"("05" ("string"), w425) -> (w424:string)
            }
            event "Kitchen Curtain 1": Value Change {
              n592 = event-data() -> ()  [unwired: 1 in, 1 out]
              n593 = Format Into String "Format Into String"(format string="%03d", "Kitchen Curtain 1") -> (resulting string=w428:string)  [unwired: 2 in, 1 out]
              n594 = Type Cast(x=w428) -> (*(type *) &x=w431:string)  [unwired: 1 in]
              n595 = Concatenate Strings "Concatenate Strings"("06" ("string"), w431) -> (w430:string)
            }
            event "Kitchen Curtain 2": Value Change {
              n596 = event-data() -> ()  [unwired: 1 in, 1 out]
              n597 = Format Into String "Format Into String"(format string="%03d", "Kitchen Curtain 2") -> (resulting string=w434:string)  [unwired: 2 in, 1 out]
              n598 = Type Cast(x=w434) -> (*(type *) &x=w437:string)  [unwired: 1 in]
              n599 = Concatenate Strings "Concatenate Strings"("07" ("string"), w437) -> (w436:string)
            }
          }
          n600 = String Length(string=w381) -> (length=w388:i32)
          n601 = Type Cast(x=w388) -> (*(type *) &x=w387:string)  [unwired: 1 in]
          n602 = TCP Write "TCP Write\nCarrying Info\nString Length"(connection ID=w384, data in=w387, error in (no error)=w385) -> (connection ID out=w389:refnum<k5>, error out=w390:errorcluster)  [unwired: 1 in, 1 out]
          n603 = TCP Write "TCP Write\nCarrying\nData"(connection ID=w389, data in=w381, error in (no error)=w390) -> (connection ID out=w382:refnum<k5>, error out=w383:errorcluster)  [unwired: 1 in, 1 out]
        }
        n604 = TCP Close Connection "TCP Close \nConnection"(connection ID=w216, error in (no error)=w217) -> (error out=w218:errorcluster)  [unwired: 1 in, 1 out]
        n605 = call <vilib>:"Clear Errors.vi"("error in (no error)"=w218) -> ()  [unwired: 5 in, 2 out]
        n606 = TCP Open Connection "TCP Open \nConnection"(address="localhost", remote port or service name=u16 51115) -> (connection ID=w194:refnum<k5>, error out=w193:errorcluster)  [unwired: 3 in]
        n607 = while "Brightness" {
          tunnel: w193 -> [w266]
          tunnel: w194 -> [w265]
          tunnel: [w264] -> w196
          tunnel: [w263] -> w197
          stop <- FALSE stop-if-true
          n608 = event shown="[1] \"Brightness Kitchen  Light 1\": Value Change" {
            selector: _ -> [_ _ _ _ _ _ _ _ _ _ _ _ _ _ _ _ _ _ _ _ _ _]
            dyn-events: _ -> [_ _ _ _ _ _ _ _ _ _ _ _ _ _ _ _ _ _ _ _ _ _]
            timeout: _ -> [_ _ _ _ _ _ _ _ _ _ _ _ _ _ _ _ _ _ _ _ _ _]
            tunnel: [w275 w280 w285 w290 w295 w300 w305 w310 w315 w320 w325 w330 w335 w340 w345 w350 w355 w360 w365 w370 w375 w377] -> w262
            event "Brightness\nMaster Bedroom \nLight 1": Value Change {
              n609 = event-data() -> ()  [unwired: 1 in, 1 out]
              n610 = Format Into String "Format Into String"(format string="%03d", "Brightness\nMaster Bedroom \nLight 1") -> (resulting string=w273:string)  [unwired: 2 in, 1 out]
              n611 = Concatenate Strings "Concatenate Strings"("00" ("string"), w273) -> (w275:string)
            }
            event "Brightness\nKitchen \nLight 1": Value Change {
              n612 = event-data() -> ()  [unwired: 1 in, 1 out]
              n613 = Format Into String "Format Into String"(format string="%03d", "Brightness\nKitchen \nLight 1") -> (resulting string=w278:string)  [unwired: 2 in, 1 out]
              n614 = Concatenate Strings "Concatenate Strings"("01" ("string"), w278) -> (w280:string)
            }
            event "Brightness\nKitchen \nLight 2": Value Change {
              n615 = event-data() -> ()  [unwired: 1 in, 1 out]
              n616 = Format Into String "Format Into String"(format string="%03d", "Brightness\nKitchen \nLight 2") -> (resulting string=w283:string)  [unwired: 2 in, 1 out]
              n617 = Concatenate Strings "Concatenate Strings"("02" ("string"), w283) -> (w285:string)
            }
            event "Brightness\nService Laundry \nLight 1": Value Change {
              n618 = event-data() -> ()  [unwired: 1 in, 1 out]
              n619 = Format Into String "Format Into String"(format string="%03d", "Brightness\nService Laundry \nLight 1") -> (resulting string=w288:string)  [unwired: 2 in, 1 out]
              n620 = Concatenate Strings "Concatenate Strings"("03" ("string"), w288) -> (w290:string)
            }
            event "Brightness\nService Laundry \nLight 2": Value Change {
              n621 = event-data() -> ()  [unwired: 1 in, 1 out]
              n622 = Format Into String "Format Into String"(format string="%03d", "Brightness\nService Laundry \nLight 2") -> (resulting string=w293:string)  [unwired: 2 in, 1 out]
              n623 = Concatenate Strings "Concatenate Strings"("04" ("string"), w293) -> (w295:string)
            }
            event "Brightness\nT&B Light": Value Change {
              n624 = event-data() -> ()  [unwired: 1 in, 1 out]
              n625 = Format Into String "Format Into String"(format string="%03d", "Brightness\nT&B Light") -> (resulting string=w298:string)  [unwired: 2 in, 1 out]
              n626 = Concatenate Strings "Concatenate Strings"("05" ("string"), w298) -> (w300:string)
            }
            event "Brightness\nMaster Bedroom \nLight 2": Value Change {
              n627 = event-data() -> ()  [unwired: 1 in, 1 out]
              n628 = Format Into String "Format Into String"(format string="%03d", "Brightness\nMaster Bedroom \nLight 2") -> (resulting string=w303:string)  [unwired: 2 in, 1 out]
              n629 = Concatenate Strings "Concatenate Strings"("06" ("string"), w303) -> (w305:string)
            }
            event "Brightness\nMaster Bedroom \nW.I.C. Light": Value Change {
              n630 = event-data() -> ()  [unwired: 1 in, 1 out]
              n631 = Format Into String "Format Into String"(format string="%03d", "Brightness\nMaster Bedroom \nW.I.C. Light") -> (resulting string=w308:string)  [unwired: 2 in, 1 out]
              n632 = Concatenate Strings "Concatenate Strings"("07" ("string"), w308) -> (w310:string)
            }
            event "Brightness\nLiving Area Light 1": Value Change {
              n633 = event-data() -> ()  [unwired: 1 in, 1 out]
              n634 = Format Into String "Format Into String"(format string="%03d", "Brightness\nLiving Area Light 1") -> (resulting string=w313:string)  [unwired: 2 in, 1 out]
              n635 = Concatenate Strings "Concatenate Strings"("08" ("string"), w313) -> (w315:string)
            }
            event "Brightness\nLiving Area Light 2": Value Change {
              n636 = event-data() -> ()  [unwired: 1 in, 1 out]
              n637 = Format Into String "Format Into String"(format string="%03d", "Brightness\nLiving Area Light 2") -> (resulting string=w318:string)  [unwired: 2 in, 1 out]
              n638 = Concatenate Strings "Concatenate Strings"("09" ("string"), w318) -> (w320:string)
            }
            event "Brightness\n Porch Light": Value Change {
              n639 = event-data() -> ()  [unwired: 1 in, 1 out]
              n640 = Format Into String "Format Into String"(format string="%03d", "Brightness\n Porch Light") -> (resulting string=w323:string)  [unwired: 2 in, 1 out]
              n641 = Concatenate Strings "Concatenate Strings"("10" ("string"), w323) -> (w325:string)
            }
            event "Brightness\nDining Area Light 1": Value Change {
              n642 = event-data() -> ()  [unwired: 1 in, 1 out]
              n643 = Format Into String "Format Into String"(format string="%03d", "Brightness\nDining Area Light 1") -> (resulting string=w328:string)  [unwired: 2 in, 1 out]
              n644 = Concatenate Strings "Concatenate Strings"("11" ("string"), w328) -> (w330:string)
            }
            event "Brightness\nDining Area Light 2": Value Change {
              n645 = event-data() -> ()  [unwired: 1 in, 1 out]
              n646 = Format Into String "Format Into String"(format string="%03d", "Brightness\nDining Area Light 2") -> (resulting string=w333:string)  [unwired: 2 in, 1 out]
              n647 = Concatenate Strings "Concatenate Strings"("12" ("string"), w333) -> (w335:string)
            }
            event "Brightness\nLanai Light": Value Change {
              n648 = event-data() -> ()  [unwired: 1 in, 1 out]
              n649 = Format Into String "Format Into String"(format string="%03d", "Brightness\nLanai Light") -> (resulting string=w338:string)  [unwired: 2 in, 1 out]
              n650 = Concatenate Strings "Concatenate Strings"("13" ("string"), w338) -> (w340:string)
            }
            event "Brightness\nBedroom 2 \nLight 1": Value Change {
              n651 = event-data() -> ()  [unwired: 1 in, 1 out]
              n652 = Format Into String "Format Into String"(format string="%03d", "Brightness\nBedroom 2 \nLight 1") -> (resulting string=w343:string)  [unwired: 2 in, 1 out]
              n653 = Concatenate Strings "Concatenate Strings"("14" ("string"), w343) -> (w345:string)
            }
            event "Brightness\nBedroom 2 \nLight 2": Value Change {
              n654 = event-data() -> ()  [unwired: 1 in, 1 out]
              n655 = Format Into String "Format Into String"(format string="%03d", "Brightness\nBedroom 2 \nLight 2") -> (resulting string=w348:string)  [unwired: 2 in, 1 out]
              n656 = Concatenate Strings "Concatenate Strings"("15" ("string"), w348) -> (w350:string)
            }
            event "Brightness\nBedroom 2 \nW.I.C. Light": Value Change {
              n657 = event-data() -> ()  [unwired: 1 in, 1 out]
              n658 = Format Into String "Format Into String"(format string="%03d", "Brightness\nBedroom 2 \nW.I.C. Light") -> (resulting string=w353:string)  [unwired: 2 in, 1 out]
              n659 = Concatenate Strings "Concatenate Strings"("16" ("string"), w353) -> (w355:string)
            }
            event "Brightness\nBedroom 3 \nLight 1": Value Change {
              n660 = event-data() -> ()  [unwired: 1 in, 1 out]
              n661 = Format Into String "Format Into String"(format string="%03d", "Brightness\nBedroom 3 \nLight 1") -> (resulting string=w358:string)  [unwired: 2 in, 1 out]
              n662 = Concatenate Strings "Concatenate Strings"("17" ("string"), w358) -> (w360:string)
            }
            event "Brightness\nBedroom 3 \nLight 2": Value Change {
              n663 = event-data() -> ()  [unwired: 1 in, 1 out]
              n664 = Format Into String "Format Into String"(format string="%03d", "Brightness\nBedroom 3 \nLight 2") -> (resulting string=w363:string)  [unwired: 2 in, 1 out]
              n665 = Concatenate Strings "Concatenate Strings"("18" ("string"), w363) -> (w365:string)
            }
            event "Brightness\nGarage Light 1": Value Change {
              n666 = event-data() -> ()  [unwired: 1 in, 1 out]
              n667 = Format Into String "Format Into String"(format string="%03d", "Brightness\nGarage Light 1") -> (resulting string=w368:string)  [unwired: 2 in, 1 out]
              n668 = Concatenate Strings "Concatenate Strings"("19" ("string"), w368) -> (w370:string)
            }
            event "Brightness\nGarage Light 2": Value Change {
              n669 = event-data() -> ()  [unwired: 1 in, 1 out]
              n670 = Format Into String "Format Into String"(format string="%03d", "Brightness\nGarage Light 2") -> (resulting string=w373:string)  [unwired: 2 in, 1 out]
              n671 = Concatenate Strings "Concatenate Strings"("20" ("string"), w373) -> (w375:string)
            }
            event "Brightness\nMaster Bath \nLight": Value Change {
              n672 = event-data() -> ()  [unwired: 1 in, 1 out]
              n673 = Format Into String "Format Into String"(format string="%03d", "Brightness\nMaster Bath \nLight") -> (resulting string=w380:string)  [unwired: 2 in, 1 out]
              n674 = Concatenate Strings "Concatenate Strings"("21" ("string"), w380) -> (w377:string)
            }
          }
          n675 = String Length(string=w262) -> (length=w268:i32)
          n676 = Type Cast(x=w268) -> (*(type *) &x=w261:string)  [unwired: 1 in]
          n677 = TCP Write "TCP Write\nCarrying Info\nString Length"(connection ID=w265, data in=w261, error in (no error)=w266) -> (connection ID out=w269:refnum<k5>, error out=w270:errorcluster)  [unwired: 1 in, 1 out]
          n678 = TCP Write "TCP Write\nCarrying\nData"(connection ID=w269, data in=w262, error in (no error)=w270) -> (connection ID out=w263:refnum<k5>, error out=w264:errorcluster)  [unwired: 1 in, 1 out]
        }
        n679 = TCP Close Connection "TCP Close \nConnection"(connection ID=w198, error in (no error)=w199) -> (error out=w200:errorcluster)  [unwired: 1 in, 1 out]
        n680 = call <vilib>:"Clear Errors.vi"("error in (no error)"=w200) -> ()  [unwired: 5 in, 2 out]
        n681 = TCP Close Connection "TCP Close \nConnection"(connection ID=w197, error in (no error)=w196) -> (error out=w195:errorcluster)  [unwired: 1 in, 1 out]
        n682 = call <vilib>:"Clear Errors.vi"("error in (no error)"=w195) -> ()  [unwired: 5 in, 2 out]
        n683 = TCP Open Connection "TCP Open \nConnection"(address="localhost", remote port or service name=u16 51116) -> (connection ID=w187:refnum<k5>, error out=w188:errorcluster)  [unwired: 3 in]
        n684 = while "Brightness" {
          tunnel: w188 -> [w240]
          tunnel: w187 -> [w239]
          tunnel: [w238] -> w185
          tunnel: [w237] -> w184
          stop <- FALSE stop-if-true
          n685 = event shown="[3] \"Living Area AirCon\": Value Change" {
            selector: _ -> [_ _ _ _]
            dyn-events: _ -> [_ _ _ _]
            timeout: _ -> [_ _ _ _]
            tunnel: [w246 w250 w254 w258] -> w235
            event "Master Bedroom AirCon": Value Change {
              n686 = event-data() -> ()  [unwired: 1 in, 6 out]
              n687 = Type Cast(x="Master Bedroom AirCon") -> (*(type *) &x=w247:string)  [unwired: 1 in]
              n688 = Concatenate Strings "Concatenate Strings"("AC1" ("string"), w247) -> (w246:string)
            }
            event "Bedroom 3 AirCon": Value Change {
              n689 = event-data() -> ()  [unwired: 1 in, 6 out]
              n690 = Type Cast(x="Bedroom 3 AirCon") -> (*(type *) &x=w251:string)  [unwired: 1 in]
              n691 = Concatenate Strings "Concatenate Strings"("AC2" ("string"), w251) -> (w250:string)
            }
            event "Bedroom 2 AirCon": Value Change {
              n692 = event-data() -> ()  [unwired: 1 in, 6 out]
              n693 = Type Cast(x="Bedroom 2 AirCon") -> (*(type *) &x=w255:string)  [unwired: 1 in]
              n694 = Concatenate Strings "Concatenate Strings"("AC3" ("string"), w255) -> (w254:string)
            }
            event "Living Area AirCon": Value Change {
              n695 = event-data() -> ()  [unwired: 1 in, 6 out]
              n696 = Type Cast(x="Living Area AirCon") -> (*(type *) &x=w259:string)  [unwired: 1 in]
              n697 = Concatenate Strings "Concatenate Strings"("AC4" ("string"), w259) -> (w258:string)
            }
          }
          n698 = String Length(string=w235) -> (length=w242:i32)
          n699 = Type Cast(x=w242) -> (*(type *) &x=w236:string)  [unwired: 1 in]
          n700 = TCP Write "TCP Write\nCarrying Info\nString Length"(connection ID=w239, data in=w236, error in (no error)=w240) -> (connection ID out=w243:refnum<k5>, error out=w244:errorcluster)  [unwired: 1 in, 1 out]
          n701 = TCP Write "TCP Write\nCarrying\nData"(connection ID=w243, data in=w235, error in (no error)=w244) -> (connection ID out=w237:refnum<k5>, error out=w238:errorcluster)  [unwired: 1 in, 1 out]
        }
        n702 = TCP Close Connection "TCP Close \nConnection"(connection ID=w184, error in (no error)=w185) -> (error out=w186:errorcluster)  [unwired: 1 in, 1 out]
        n703 = call <vilib>:"Clear Errors.vi"("error in (no error)"=w186) -> ()  [unwired: 5 in, 2 out]
      }
    }
  }
  n704 = while {
    stop <- FALSE stop-if-true
    n705 = Get Date/Time In Seconds() -> (seconds since 1Jan1904=→"Current Time":timestamp)
  }
  "Login" <- FALSE ("Status 2")
